vi "MultirunBuilderForNamedLocations.vi"() -> ()   [LabVIEW 2015]
uses:
  Anemometry Sub Vis/Gen Trav/Spacing.ctl
  Anemometry Sub Vis/Controls/Multi_run_mode.ctl
  Anemometry Sub Vis/File/Setup_Filetype.ctl
  Anemometry Sub Vis/Globals/Meas_global.vi
panel:
  in  "Vert.Z-Locations 2":dbl[](array[numeric])=[12.7, 19.05, 25.4]
  in  "TaskArray":T3(array[cluster])=[{"Start X"=-3390.0, "Start Y"=-113.0, "Start Z"=780.0, "End X"=-3390.0, "End Y"=-113.0, "End Z"=780.0, "No. of pts."=0, "Spacing"=enum."Linear", "Filename"=path "", "Tunnel Speed"=7.64, "Averaging time (min)"=0.0, "Extra Commands"="", "Carrier_1 Q (l/min)"=0.0, "Carrier_2 Q (l/min)"=0.0, "Trace Gas Concentration (%)"=0.0, "Specific Arguments"="", "Comments"="Tunnel Warm Up", "Row No"=0, "Row Type Selector"=enum."Set Tunnel Speed Only", "Completion time"="", "Row Duration (mins)"=10.0, "No. of Valid pts."=0, "Meas Setup File"=""}, {"Start X"=-3390.0, "Start Y"=-113.0, "Start Z"=780.0, "End X"=-3390.0, "End Y"=-113.0, "End Z"=780.0, "No. of pts."=0, "Spacing"=enum."Linear", "Filename"=path "", "Tunnel Speed"=7.64, "Averaging time (min)"=0.0, "Extra Commands"="", "Carrier_1 Q (l/min)"=0.0, "Carrier_2 Q (l/min)"=0.0, "Trace Gas Concentration (%)"=0.0, "Specific Arguments"="10", "Comments"="Tunnel Warm Up", "Row No"=0, "Row Type Selector"=enum."Wait (minutes)", "Completion time"="", "Row Duration (mins)"=0.0, "No. of Valid pts."=0, "Meas Setup File"=""}, {"Start X"=0.0, "Start Y"=0.0, "Start Z"=150.0, "End X"=0.0, "End Y"=0.0, "End Z"=150.0, "No. of pts."=0, "Spacing"=enum."Linear", "Filename"=path "", "Tunnel Speed"=7.64, "Averaging time (min)"=0.0, "Extra Commands"="!Work in Tunnel Coordinates", "Carrier_1 Q (l/min)"=0.0, "Carrier_2 Q (l/min)"=0.0, "Trace Gas Concentration (%)"=0.0, "Specific Arguments"="", "Comments"="", "Row No"=0, "Row Type Selector"=enum."Move Traverse Only", "Completion time"="", "Row Duration (mins)"=0.0, "No. of Valid pts."=0, "Meas Setup File"=""}, {"Start X"=0.0, "Start Y"=0.0, "Start Z"=805.0, "End X"=0.0, "End Y"=0.0, "End Z"=805.0, "No. of pts."=0, "Spacing"=enum."Linear", "Filename"=path "", "Tunnel Speed"=7.64, "Averaging time (min)"=0.0, "Extra Commands"="!Work in Tunnel Coordinates", "Carrier_1 Q (l/min)"=0.0, "Carrier_2 Q (l/min)"=0.0, "Trace Gas Concentration (%)"=0.0, "Specific Arguments"="MoveTT.vi;10", "Comments"="", "Row No"=0, "Row Type Selector"=enum."Run VI Named:", "Completion time"="", "Row Duration (mins)"=0.0, "No. of Valid pts."=0, "Meas Setup File"=""}, {"Start X"=-72.9, "Start Y"=-56.5, "Start Z"=12.7, "End X"=-72.9, "End Y"=-56.5, "End Z"=25.4, "No. of pts."=3, "Spacing"=enum."Specified", "Filename"=path "M:/\\Projects\\8773\\Results\\Tunnel1\\AnemometerSurvey.xls", "Tunnel Speed"=7.64, "Averaging time (min)"=1.0, "Extra Commands"="", "Carrier_1 Q (l/min)"=0.0, "Carrier_2 Q (l/min)"=0.0, "Trace Gas Concentration (%)"=0.0, "Specific Arguments"="Z= ;12.7;19.1;25.4\r", "Comments"="Anemo1", "Row No"=0, "Row Type Selector"=enum."Vertical Profile", "Completion time"="", "Row Duration (mins)"=0.0, "No. of Valid pts."=0, "Meas Setup File"="Current_Setup.xls"}, {"Start X"=-458.4, "Start Y"=87.9, "Start Z"=25.6, "End X"=-458.4, "End Y"=87.9, "End Z"=38.3, "No. of pts."=3, "Spacing"=enum."Specified", "Filename"=path "M:/\\Projects\\8773\\Results\\Tunnel1\\AnemometerSurvey.xls", "Tunnel Speed"=7.64, "Averaging time (min)"=1.0, "Extra Commands"="", "Carrier_1 Q (l/min)"=0.0, "Carrier_2 Q (l/min)"=0.0, "Trace Gas Concentration (%)"=0.0, "Specific Arguments"="Z= ;25.6;32.0;38.3\r", "Comments"="Anemo2", "Row No"=0, "Row Type Selector"=enum."Vertical Profile", "Completion time"="", "Row Duration (mins)"=0.0, "No. of Valid pts."=0, "Meas Setup File"="Current_Setup.xls"}, {"Start X"=0.0, "Start Y"=0.0, "Start Z"=150.0, "End X"=0.0, "End Y"=0.0, "End Z"=150.0, "No. of pts."=0, "Spacing"=enum."Linear", "Filename"=path "", "Tunnel Speed"=7.64, "Averaging time (min)"=0.0, "Extra Commands"="!Work in Tunnel Coordinates", "Carrier_1 Q (l/min)"=0.0, "Carrier_2 Q (l/min)"=0.0, "Trace Gas Concentration (%)"=0.0, "Specific Arguments"="", "Comments"="", "Row No"=0, "Row Type Selector"=enum."Move Traverse Only", "Completion time"="", "Row Duration (mins)"=0.0, "No. of Valid pts."=0, "Meas Setup File"=""}, {"Start X"=0.0, "Start Y"=0.0, "Start Z"=805.0, "End X"=0.0, "End Y"=0.0, "End Z"=805.0, "No. of pts."=0, "Spacing"=enum."Linear", "Filename"=path "", "Tunnel Speed"=7.64, "Averaging time (min)"=0.0, "Extra Commands"="!Work in Tunnel Coordinates", "Carrier_1 Q (l/min)"=0.0, "Carrier_2 Q (l/min)"=0.0, "Trace Gas Concentration (%)"=0.0, "Specific Arguments"="MoveTT.vi;30", "Comments"="", "Row No"=0, "Row Type Selector"=enum."Run VI Named:", "Completion time"="", "Row Duration (mins)"=0.0, "No. of Valid pts."=0, "Meas Setup File"=""}, {"Start X"=-72.9, "Start Y"=-56.5, "Start Z"=12.7, "End X"=-72.9, "End Y"=-56.5, "End Z"=25.4, "No. of pts."=3, "Spacing"=enum."Specified", "Filename"=path "M:/\\Projects\\8773\\Results\\Tunnel1\\AnemometerSurvey.xls", "Tunnel Speed"=7.64, "Averaging time (min)"=1.0, "Extra Commands"="", "Carrier_1 Q (l/min)"=0.0, "Carrier_2 Q (l/min)"=0.0, "Trace Gas Concentration (%)"=0.0, "Specific Arguments"="Z= ;12.7;19.1;25.4\r", "Comments"="Anemo1", "Row No"=0, "Row Type Selector"=enum."Vertical Profile", "Completion time"="", "Row Duration (mins)"=0.0, "No. of Valid pts."=0, "Meas Setup File"="Current_Setup.xls"}, {"Start X"=-458.4, "Start Y"=87.9, "Start Z"=25.6, "End X"=-458.4, "End Y"=87.9, "End Z"=38.3, "No. of pts."=3, "Spacing"=enum."Specified", "Filename"=path "M:/\\Projects\\8773\\Results\\Tunnel1\\AnemometerSurvey.xls", "Tunnel Speed"=7.64, "Averaging time (min)"=1.0, "Extra Commands"="", "Carrier_1 Q (l/min)"=0.0, "Carrier_2 Q (l/min)"=0.0, "Trace Gas Concentration (%)"=0.0, "Specific Arguments"="Z= ;25.6;32.0;38.3\r", "Comments"="Anemo2", "Row No"=0, "Row Type Selector"=enum."Vertical Profile", "Completion time"="", "Row Duration (mins)"=0.0, "No. of Valid pts."=0, "Meas Setup File"="Current_Setup.xls"}, {"Start X"=0.0, "Start Y"=0.0, "Start Z"=150.0, "End X"=0.0, "End Y"=0.0, "End Z"=150.0, "No. of pts."=0, "Spacing"=enum."Linear", "Filename"=path "", "Tunnel Speed"=7.64, "Averaging time (min)"=0.0, "Extra Commands"="!Work in Tunnel Coordinates", "Carrier_1 Q (l/min)"=0.0, "Carrier_2 Q (l/min)"=0.0, "Trace Gas Concentration (%)"=0.0, "Specific Arguments"="", "Comments"="", "Row No"=0, "Row Type Selector"=enum."Move Traverse Only", "Completion time"="", "Row Duration (mins)"=0.0, "No. of Valid pts."=0, "Meas Setup File"=""}, {"Start X"=0.0, "Start Y"=0.0, "Start Z"=805.0, "End X"=0.0, "End Y"=0.0, "End Z"=805.0, "No. of pts."=0, "Spacing"=enum."Linear", "Filename"=path "", "Tunnel Speed"=7.64, "Averaging time (min)"=0.0, "Extra Commands"="!Work in Tunnel Coordinates", "Carrier_1 Q (l/min)"=0.0, "Carrier_2 Q (l/min)"=0.0, "Trace Gas Concentration (%)"=0.0, "Specific Arguments"="MoveTT.vi;50", "Comments"="", "Row No"=0, "Row Type Selector"=enum."Run VI Named:", "Completion time"="", "Row Duration (mins)"=0.0, "No. of Valid pts."=0, "Meas Setup File"=""}, {"Start X"=-72.9, "Start Y"=-56.5, "Start Z"=12.7, "End X"=-72.9, "End Y"=-56.5, "End Z"=25.4, "No. of pts."=3, "Spacing"=enum."Specified", "Filename"=path "M:/\\Projects\\8773\\Results\\Tunnel1\\AnemometerSurvey.xls", "Tunnel Speed"=7.64, "Averaging time (min)"=1.0, "Extra Commands"="", "Carrier_1 Q (l/min)"=0.0, "Carrier_2 Q (l/min)"=0.0, "Trace Gas Concentration (%)"=0.0, "Specific Arguments"="Z= ;12.7;19.1;25.4\r", "Comments"="Anemo1", "Row No"=0, "Row Type Selector"=enum."Vertical Profile", "Completion time"="", "Row Duration (mins)"=0.0, "No. of Valid pts."=0, "Meas Setup File"="Current_Setup.xls"}, {"Start X"=-458.4, "Start Y"=87.9, "Start Z"=25.6, "End X"=-458.4, "End Y"=87.9, "End Z"=38.3, "No. of pts."=3, "Spacing"=enum."Specified", "Filename"=path "M:/\\Projects\\8773\\Results\\Tunnel1\\AnemometerSurvey.xls", "Tunnel Speed"=7.64, "Averaging time (min)"=1.0, "Extra Commands"="", "Carrier_1 Q (l/min)"=0.0, "Carrier_2 Q (l/min)"=0.0, "Trace Gas Concentration (%)"=0.0, "Specific Arguments"="Z= ;25.6;32.0;38.3\r", "Comments"="Anemo2", "Row No"=0, "Row Type Selector"=enum."Vertical Profile", "Completion time"="", "Row Duration (mins)"=0.0, "No. of Valid pts."=0, "Meas Setup File"="Current_Setup.xls"}, {"Start X"=0.0, "Start Y"=0.0, "Start Z"=150.0, "End X"=0.0, "End Y"=0.0, "End Z"=150.0, "No. of pts."=0, "Spacing"=enum."Linear", "Filename"=path "", "Tunnel Speed"=7.64, "Averaging time (min)"=0.0, "Extra Commands"="!Work in Tunnel Coordinates", "Carrier_1 Q (l/min)"=0.0, "Carrier_2 Q (l/min)"=0.0, "Trace Gas Concentration (%)"=0.0, "Specific Arguments"="", "Comments"="", "Row No"=0, "Row Type Selector"=enum."Move Traverse Only", "Completion time"="", "Row Duration (mins)"=0.0, "No. of Valid pts."=0, "Meas Setup File"=""}, {"Start X"=0.0, "Start Y"=0.0, "Start Z"=805.0, "End X"=0.0, "End Y"=0.0, "End Z"=805.0, "No. of pts."=0, "Spacing"=enum."Linear", "Filename"=path "", "Tunnel Speed"=7.64, "Averaging time (min)"=0.0, "Extra Commands"="!Work in Tunnel Coordinates", "Carrier_1 Q (l/min)"=0.0, "Carrier_2 Q (l/min)"=0.0, "Trace Gas Concentration (%)"=0.0, "Specific Arguments"="MoveTT.vi;70", "Comments"="", "Row No"=0, "Row Type Selector"=enum."Run VI Named:", "Completion time"="", "Row Duration (mins)"=0.0, "No. of Valid pts."=0, "Meas Setup File"=""}, {"Start X"=-72.9, "Start Y"=-56.5, "Start Z"=12.7, "End X"=-72.9, "End Y"=-56.5, "End Z"=25.4, "No. of pts."=3, "Spacing"=enum."Specified", "Filename"=path "M:/\\Projects\\8773\\Results\\Tunnel1\\AnemometerSurvey.xls", "Tunnel Speed"=7.64, "Averaging time (min)"=1.0, "Extra Commands"="", "Carrier_1 Q (l/min)"=0.0, "Carrier_2 Q (l/min)"=0.0, "Trace Gas Concentration (%)"=0.0, "Specific Arguments"="Z= ;12.7;19.1;25.4\r", "Comments"="Anemo1", "Row No"=0, "Row Type Selector"=enum."Vertical Profile", "Completion time"="", "Row Duration (mins)"=0.0, "No. of Valid pts."=0, "Meas Setup File"="Current_Setup.xls"}, {"Start X"=-458.4, "Start Y"=87.9, "Start Z"=25.6, "End X"=-458.4, "End Y"=87.9, "End Z"=38.3, "No. of pts."=3, "Spacing"=enum."Specified", "Filename"=path "M:/\\Projects\\8773\\Results\\Tunnel1\\AnemometerSurvey.xls", "Tunnel Speed"=7.64, "Averaging time (min)"=1.0, "Extra Commands"="", "Carrier_1 Q (l/min)"=0.0, "Carrier_2 Q (l/min)"=0.0, "Trace Gas Concentration (%)"=0.0, "Specific Arguments"="Z= ;25.6;32.0;38.3\r", "Comments"="Anemo2", "Row No"=0, "Row Type Selector"=enum."Vertical Profile", "Completion time"="", "Row Duration (mins)"=0.0, "No. of Valid pts."=0, "Meas Setup File"="Current_Setup.xls"}, {"Start X"=0.0, "Start Y"=0.0, "Start Z"=150.0, "End X"=0.0, "End Y"=0.0, "End Z"=150.0, "No. of pts."=0, "Spacing"=enum."Linear", "Filename"=path "", "Tunnel Speed"=7.64, "Averaging time (min)"=0.0, "Extra Commands"="!Work in Tunnel Coordinates", "Carrier_1 Q (l/min)"=0.0, "Carrier_2 Q (l/min)"=0.0, "Trace Gas Concentration (%)"=0.0, "Specific Arguments"="", "Comments"="", "Row No"=0, "Row Type Selector"=enum."Move Traverse Only", "Completion time"="", "Row Duration (mins)"=0.0, "No. of Valid pts."=0, "Meas Setup File"=""}, {"Start X"=0.0, "Start Y"=0.0, "Start Z"=805.0, "End X"=0.0, "End Y"=0.0, "End Z"=805.0, "No. of pts."=0, "Spacing"=enum."Linear", "Filename"=path "", "Tunnel Speed"=7.64, "Averaging time (min)"=0.0, "Extra Commands"="!Work in Tunnel Coordinates", "Carrier_1 Q (l/min)"=0.0, "Carrier_2 Q (l/min)"=0.0, "Trace Gas Concentration (%)"=0.0, "Specific Arguments"="MoveTT.vi;90", "Comments"="", "Row No"=0, "Row Type Selector"=enum."Run VI Named:", "Completion time"="", "Row Duration (mins)"=0.0, "No. of Valid pts."=0, "Meas Setup File"=""}, {"Start X"=-72.9, "Start Y"=-56.5, "Start Z"=12.7, "End X"=-72.9, "End Y"=-56.5, "End Z"=25.4, "No. of pts."=3, "Spacing"=enum."Specified", "Filename"=path "M:/\\Projects\\8773\\Results\\Tunnel1\\AnemometerSurvey.xls", "Tunnel Speed"=7.64, "Averaging time (min)"=1.0, "Extra Commands"="", "Carrier_1 Q (l/min)"=0.0, "Carrier_2 Q (l/min)"=0.0, "Trace Gas Concentration (%)"=0.0, "Specific Arguments"="Z= ;12.7;19.1;25.4\r", "Comments"="Anemo1", "Row No"=0, "Row Type Selector"=enum."Vertical Profile", "Completion time"="", "Row Duration (mins)"=0.0, "No. of Valid pts."=0, "Meas Setup File"="Current_Setup.xls"}, {"Start X"=-458.4, "Start Y"=87.9, "Start Z"=25.6, "End X"=-458.4, "End Y"=87.9, "End Z"=38.3, "No. of pts."=3, "Spacing"=enum."Specified", "Filename"=path "M:/\\Projects\\8773\\Results\\Tunnel1\\AnemometerSurvey.xls", "Tunnel Speed"=7.64, "Averaging time (min)"=1.0, "Extra Commands"="", "Carrier_1 Q (l/min)"=0.0, "Carrier_2 Q (l/min)"=0.0, "Trace Gas Concentration (%)"=0.0, "Specific Arguments"="Z= ;25.6;32.0;38.3\r", "Comments"="Anemo2", "Row No"=0, "Row Type Selector"=enum."Vertical Profile", "Completion time"="", "Row Duration (mins)"=0.0, "No. of Valid pts."=0, "Meas Setup File"="Current_Setup.xls"}, {"Start X"=0.0, "Start Y"=0.0, "Start Z"=150.0, "End X"=0.0, "End Y"=0.0, "End Z"=150.0, "No. of pts."=0, "Spacing"=enum."Linear", "Filename"=path "", "Tunnel Speed"=7.64, "Averaging time (min)"=0.0, "Extra Commands"="!Work in Tunnel Coordinates", "Carrier_1 Q (l/min)"=0.0, "Carrier_2 Q (l/min)"=0.0, "Trace Gas Concentration (%)"=0.0, "Specific Arguments"="", "Comments"="", "Row No"=0, "Row Type Selector"=enum."Move Traverse Only", "Completion time"="", "Row Duration (mins)"=0.0, "No. of Valid pts."=0, "Meas Setup File"=""}, {"Start X"=0.0, "Start Y"=0.0, "Start Z"=805.0, "End X"=0.0, "End Y"=0.0, "End Z"=805.0, "No. of pts."=0, "Spacing"=enum."Linear", "Filename"=path "", "Tunnel Speed"=7.64, "Averaging time (min)"=0.0, "Extra Commands"="!Work in Tunnel Coordinates", "Carrier_1 Q (l/min)"=0.0, "Carrier_2 Q (l/min)"=0.0, "Trace Gas Concentration (%)"=0.0, "Specific Arguments"="MoveTT.vi;110", "Comments"="", "Row No"=0, "Row Type Selector"=enum."Run VI Named:", "Completion time"="", "Row Duration (mins)"=0.0, "No. of Valid pts."=0, "Meas Setup File"=""}, {"Start X"=-72.9, "Start Y"=-56.5, "Start Z"=12.7, "End X"=-72.9, "End Y"=-56.5, "End Z"=25.4, "No. of pts."=3, "Spacing"=enum."Specified", "Filename"=path "M:/\\Projects\\8773\\Results\\Tunnel1\\AnemometerSurvey.xls", "Tunnel Speed"=7.64, "Averaging time (min)"=1.0, "Extra Commands"="", "Carrier_1 Q (l/min)"=0.0, "Carrier_2 Q (l/min)"=0.0, "Trace Gas Concentration (%)"=0.0, "Specific Arguments"="Z= ;12.7;19.1;25.4\r", "Comments"="Anemo1", "Row No"=0, "Row Type Selector"=enum."Vertical Profile", "Completion time"="", "Row Duration (mins)"=0.0, "No. of Valid pts."=0, "Meas Setup File"="Current_Setup.xls"}, {"Start X"=-458.4, "Start Y"=87.9, "Start Z"=25.6, "End X"=-458.4, "End Y"=87.9, "End Z"=38.3, "No. of pts."=3, "Spacing"=enum."Specified", "Filename"=path "M:/\\Projects\\8773\\Results\\Tunnel1\\AnemometerSurvey.xls", "Tunnel Speed"=7.64, "Averaging time (min)"=1.0, "Extra Commands"="", "Carrier_1 Q (l/min)"=0.0, "Carrier_2 Q (l/min)"=0.0, "Trace Gas Concentration (%)"=0.0, "Specific Arguments"="Z= ;25.6;32.0;38.3\r", "Comments"="Anemo2", "Row No"=0, "Row Type Selector"=enum."Vertical Profile", "Completion time"="", "Row Duration (mins)"=0.0, "No. of Valid pts."=0, "Meas Setup File"="Current_Setup.xls"}, {"Start X"=0.0, "Start Y"=0.0, "Start Z"=150.0, "End X"=0.0, "End Y"=0.0, "End Z"=150.0, "No. of pts."=0, "Spacing"=enum."Linear", "Filename"=path "", "Tunnel Speed"=7.64, "Averaging time (min)"=0.0, "Extra Commands"="!Work in Tunnel Coordinates", "Carrier_1 Q (l/min)"=0.0, "Carrier_2 Q (l/min)"=0.0, "Trace Gas Concentration (%)"=0.0, "Specific Arguments"="", "Comments"="", "Row No"=0, "Row Type Selector"=enum."Move Traverse Only", "Completion time"="", "Row Duration (mins)"=0.0, "No. of Valid pts."=0, "Meas Setup File"=""}, {"Start X"=0.0, "Start Y"=0.0, "Start Z"=805.0, "End X"=0.0, "End Y"=0.0, "End Z"=805.0, "No. of pts."=0, "Spacing"=enum."Linear", "Filename"=path "", "Tunnel Speed"=7.64, "Averaging time (min)"=0.0, "Extra Commands"="!Work in Tunnel Coordinates", "Carrier_1 Q (l/min)"=0.0, "Carrier_2 Q (l/min)"=0.0, "Trace Gas Concentration (%)"=0.0, "Specific Arguments"="MoveTT.vi;130", "Comments"="", "Row No"=0, "Row Type Selector"=enum."Run VI Named:", "Completion time"="", "Row Duration (mins)"=0.0, "No. of Valid pts."=0, "Meas Setup File"=""}, {"Start X"=-72.9, "Start Y"=-56.5, "Start Z"=12.7, "End X"=-72.9, "End Y"=-56.5, "End Z"=25.4, "No. of pts."=3, "Spacing"=enum."Specified", "Filename"=path "M:/\\Projects\\8773\\Results\\Tunnel1\\AnemometerSurvey.xls", "Tunnel Speed"=7.64, "Averaging time (min)"=1.0, "Extra Commands"="", "Carrier_1 Q (l/min)"=0.0, "Carrier_2 Q (l/min)"=0.0, "Trace Gas Concentration (%)"=0.0, "Specific Arguments"="Z= ;12.7;19.1;25.4\r", "Comments"="Anemo1", "Row No"=0, "Row Type Selector"=enum."Vertical Profile", "Completion time"="", "Row Duration (mins)"=0.0, "No. of Valid pts."=0, "Meas Setup File"="Current_Setup.xls"}, {"Start X"=-458.4, "Start Y"=87.9, "Start Z"=25.6, "End X"=-458.4, "End Y"=87.9, "End Z"=38.3, "No. of pts."=3, "Spacing"=enum."Specified", "Filename"=path "M:/\\Projects\\8773\\Results\\Tunnel1\\AnemometerSurvey.xls", "Tunnel Speed"=7.64, "Averaging time (min)"=1.0, "Extra Commands"="", "Carrier_1 Q (l/min)"=0.0, "Carrier_2 Q (l/min)"=0.0, "Trace Gas Concentration (%)"=0.0, "Specific Arguments"="Z= ;25.6;32.0;38.3\r", "Comments"="Anemo2", "Row No"=0, "Row Type Selector"=enum."Vertical Profile", "Completion time"="", "Row Duration (mins)"=0.0, "No. of Valid pts."=0, "Meas Setup File"="Current_Setup.xls"}, {"Start X"=0.0, "Start Y"=0.0, "Start Z"=150.0, "End X"=0.0, "End Y"=0.0, "End Z"=150.0, "No. of pts."=0, "Spacing"=enum."Linear", "Filename"=path "", "Tunnel Speed"=7.64, "Averaging time (min)"=0.0, "Extra Commands"="!Work in Tunnel Coordinates", "Carrier_1 Q (l/min)"=0.0, "Carrier_2 Q (l/min)"=0.0, "Trace Gas Concentration (%)"=0.0, "Specific Arguments"="", "Comments"="", "Row No"=0, "Row Type Selector"=enum."Move Traverse Only", "Completion time"="", "Row Duration (mins)"=0.0, "No. of Valid pts."=0, "Meas Setup File"=""}, {"Start X"=0.0, "Start Y"=0.0, "Start Z"=805.0, "End X"=0.0, "End Y"=0.0, "End Z"=805.0, "No. of pts."=0, "Spacing"=enum."Linear", "Filename"=path "", "Tunnel Speed"=7.64, "Averaging time (min)"=0.0, "Extra Commands"="!Work in Tunnel Coordinates", "Carrier_1 Q (l/min)"=0.0, "Carrier_2 Q (l/min)"=0.0, "Trace Gas Concentration (%)"=0.0, "Specific Arguments"="MoveTT.vi;150", "Comments"="", "Row No"=0, "Row Type Selector"=enum."Run VI Named:", "Completion time"="", "Row Duration (mins)"=0.0, "No. of Valid pts."=0, "Meas Setup File"=""}, {"Start X"=-72.9, "Start Y"=-56.5, "Start Z"=12.7, "End X"=-72.9, "End Y"=-56.5, "End Z"=25.4, "No. of pts."=3, "Spacing"=enum."Specified", "Filename"=path "M:/\\Projects\\8773\\Results\\Tunnel1\\AnemometerSurvey.xls", "Tunnel Speed"=7.64, "Averaging time (min)"=1.0, "Extra Commands"="", "Carrier_1 Q (l/min)"=0.0, "Carrier_2 Q (l/min)"=0.0, "Trace Gas Concentration (%)"=0.0, "Specific Arguments"="Z= ;12.7;19.1;25.4\r", "Comments"="Anemo1", "Row No"=0, "Row Type Selector"=enum."Vertical Profile", "Completion time"="", "Row Duration (mins)"=0.0, "No. of Valid pts."=0, "Meas Setup File"="Current_Setup.xls"}, {"Start X"=-458.4, "Start Y"=87.9, "Start Z"=25.6, "End X"=-458.4, "End Y"=87.9, "End Z"=38.3, "No. of pts."=3, "Spacing"=enum."Specified", "Filename"=path "M:/\\Projects\\8773\\Results\\Tunnel1\\AnemometerSurvey.xls", "Tunnel Speed"=7.64, "Averaging time (min)"=1.0, "Extra Commands"="", "Carrier_1 Q (l/min)"=0.0, "Carrier_2 Q (l/min)"=0.0, "Trace Gas Concentration (%)"=0.0, "Specific Arguments"="Z= ;25.6;32.0;38.3\r", "Comments"="Anemo2", "Row No"=0, "Row Type Selector"=enum."Vertical Profile", "Completion time"="", "Row Duration (mins)"=0.0, "No. of Valid pts."=0, "Meas Setup File"="Current_Setup.xls"}, {"Start X"=0.0, "Start Y"=0.0, "Start Z"=150.0, "End X"=0.0, "End Y"=0.0, "End Z"=150.0, "No. of pts."=0, "Spacing"=enum."Linear", "Filename"=path "", "Tunnel Speed"=7.64, "Averaging time (min)"=0.0, "Extra Commands"="!Work in Tunnel Coordinates", "Carrier_1 Q (l/min)"=0.0, "Carrier_2 Q (l/min)"=0.0, "Trace Gas Concentration (%)"=0.0, "Specific Arguments"="", "Comments"="", "Row No"=0, "Row Type Selector"=enum."Move Traverse Only", "Completion time"="", "Row Duration (mins)"=0.0, "No. of Valid pts."=0, "Meas Setup File"=""}, {"Start X"=0.0, "Start Y"=0.0, "Start Z"=805.0, "End X"=0.0, "End Y"=0.0, "End Z"=805.0, "No. of pts."=0, "Spacing"=enum."Linear", "Filename"=path "", "Tunnel Speed"=7.64, "Averaging time (min)"=0.0, "Extra Commands"="!Work in Tunnel Coordinates", "Carrier_1 Q (l/min)"=0.0, "Carrier_2 Q (l/min)"=0.0, "Trace Gas Concentration (%)"=0.0, "Specific Arguments"="MoveTT.vi;170", "Comments"="", "Row No"=0, "Row Type Selector"=enum."Run VI Named:", "Completion time"="", "Row Duration (mins)"=0.0, "No. of Valid pts."=0, "Meas Setup File"=""}, {"Start X"=-72.9, "Start Y"=-56.5, "Start Z"=12.7, "End X"=-72.9, "End Y"=-56.5, "End Z"=25.4, "No. of pts."=3, "Spacing"=enum."Specified", "Filename"=path "M:/\\Projects\\8773\\Results\\Tunnel1\\AnemometerSurvey.xls", "Tunnel Speed"=7.64, "Averaging time (min)"=1.0, "Extra Commands"="", "Carrier_1 Q (l/min)"=0.0, "Carrier_2 Q (l/min)"=0.0, "Trace Gas Concentration (%)"=0.0, "Specific Arguments"="Z= ;12.7;19.1;25.4\r", "Comments"="Anemo1", "Row No"=0, "Row Type Selector"=enum."Vertical Profile", "Completion time"="", "Row Duration (mins)"=0.0, "No. of Valid pts."=0, "Meas Setup File"="Current_Setup.xls"}, {"Start X"=-458.4, "Start Y"=87.9, "Start Z"=25.6, "End X"=-458.4, "End Y"=87.9, "End Z"=38.3, "No. of pts."=3, "Spacing"=enum."Specified", "Filename"=path "M:/\\Projects\\8773\\Results\\Tunnel1\\AnemometerSurvey.xls", "Tunnel Speed"=7.64, "Averaging time (min)"=1.0, "Extra Commands"="", "Carrier_1 Q (l/min)"=0.0, "Carrier_2 Q (l/min)"=0.0, "Trace Gas Concentration (%)"=0.0, "Specific Arguments"="Z= ;25.6;32.0;38.3\r", "Comments"="Anemo2", "Row No"=0, "Row Type Selector"=enum."Vertical Profile", "Completion time"="", "Row Duration (mins)"=0.0, "No. of Valid pts."=0, "Meas Setup File"="Current_Setup.xls"}, {"Start X"=0.0, "Start Y"=0.0, "Start Z"=150.0, "End X"=0.0, "End Y"=0.0, "End Z"=150.0, "No. of pts."=0, "Spacing"=enum."Linear", "Filename"=path "", "Tunnel Speed"=7.64, "Averaging time (min)"=0.0, "Extra Commands"="!Work in Tunnel Coordinates", "Carrier_1 Q (l/min)"=0.0, "Carrier_2 Q (l/min)"=0.0, "Trace Gas Concentration (%)"=0.0, "Specific Arguments"="", "Comments"="", "Row No"=0, "Row Type Selector"=enum."Move Traverse Only", "Completion time"="", "Row Duration (mins)"=0.0, "No. of Valid pts."=0, "Meas Setup File"=""}, {"Start X"=0.0, "Start Y"=0.0, "Start Z"=805.0, "End X"=0.0, "End Y"=0.0, "End Z"=805.0, "No. of pts."=0, "Spacing"=enum."Linear", "Filename"=path "", "Tunnel Speed"=7.64, "Averaging time (min)"=0.0, "Extra Commands"="!Work in Tunnel Coordinates", "Carrier_1 Q (l/min)"=0.0, "Carrier_2 Q (l/min)"=0.0, "Trace Gas Concentration (%)"=0.0, "Specific Arguments"="MoveTT.vi;190", "Comments"="", "Row No"=0, "Row Type Selector"=enum."Run VI Named:", "Completion time"="", "Row Duration (mins)"=0.0, "No. of Valid pts."=0, "Meas Setup File"=""}, {"Start X"=-72.9, "Start Y"=-56.5, "Start Z"=12.7, "End X"=-72.9, "End Y"=-56.5, "End Z"=25.4, "No. of pts."=3, "Spacing"=enum."Specified", "Filename"=path "M:/\\Projects\\8773\\Results\\Tunnel1\\AnemometerSurvey.xls", "Tunnel Speed"=7.64, "Averaging time (min)"=1.0, "Extra Commands"="", "Carrier_1 Q (l/min)"=0.0, "Carrier_2 Q (l/min)"=0.0, "Trace Gas Concentration (%)"=0.0, "Specific Arguments"="Z= ;12.7;19.1;25.4\r", "Comments"="Anemo1", "Row No"=0, "Row Type Selector"=enum."Vertical Profile", "Completion time"="", "Row Duration (mins)"=0.0, "No. of Valid pts."=0, "Meas Setup File"="Current_Setup.xls"}, {"Start X"=-458.4, "Start Y"=87.9, "Start Z"=25.6, "End X"=-458.4, "End Y"=87.9, "End Z"=38.3, "No. of pts."=3, "Spacing"=enum."Specified", "Filename"=path "M:/\\Projects\\8773\\Results\\Tunnel1\\AnemometerSurvey.xls", "Tunnel Speed"=7.64, "Averaging time (min)"=1.0, "Extra Commands"="", "Carrier_1 Q (l/min)"=0.0, "Carrier_2 Q (l/min)"=0.0, "Trace Gas Concentration (%)"=0.0, "Specific Arguments"="Z= ;25.6;32.0;38.3\r", "Comments"="Anemo2", "Row No"=0, "Row Type Selector"=enum."Vertical Profile", "Completion time"="", "Row Duration (mins)"=0.0, "No. of Valid pts."=0, "Meas Setup File"="Current_Setup.xls"}, {"Start X"=0.0, "Start Y"=0.0, "Start Z"=150.0, "End X"=0.0, "End Y"=0.0, "End Z"=150.0, "No. of pts."=0, "Spacing"=enum."Linear", "Filename"=path "", "Tunnel Speed"=7.64, "Averaging time (min)"=0.0, "Extra Commands"="!Work in Tunnel Coordinates", "Carrier_1 Q (l/min)"=0.0, "Carrier_2 Q (l/min)"=0.0, "Trace Gas Concentration (%)"=0.0, "Specific Arguments"="", "Comments"="", "Row No"=0, "Row Type Selector"=enum."Move Traverse Only", "Completion time"="", "Row Duration (mins)"=0.0, "No. of Valid pts."=0, "Meas Setup File"=""}, {"Start X"=0.0, "Start Y"=0.0, "Start Z"=805.0, "End X"=0.0, "End Y"=0.0, "End Z"=805.0, "No. of pts."=0, "Spacing"=enum."Linear", "Filename"=path "", "Tunnel Speed"=7.64, "Averaging time (min)"=0.0, "Extra Commands"="!Work in Tunnel Coordinates", "Carrier_1 Q (l/min)"=0.0, "Carrier_2 Q (l/min)"=0.0, "Trace Gas Concentration (%)"=0.0, "Specific Arguments"="MoveTT.vi;210", "Comments"="", "Row No"=0, "Row Type Selector"=enum."Run VI Named:", "Completion time"="", "Row Duration (mins)"=0.0, "No. of Valid pts."=0, "Meas Setup File"=""}, {"Start X"=-72.9, "Start Y"=-56.5, "Start Z"=12.7, "End X"=-72.9, "End Y"=-56.5, "End Z"=25.4, "No. of pts."=3, "Spacing"=enum."Specified", "Filename"=path "M:/\\Projects\\8773\\Results\\Tunnel1\\AnemometerSurvey.xls", "Tunnel Speed"=7.64, "Averaging time (min)"=1.0, "Extra Commands"="", "Carrier_1 Q (l/min)"=0.0, "Carrier_2 Q (l/min)"=0.0, "Trace Gas Concentration (%)"=0.0, "Specific Arguments"="Z= ;12.7;19.1;25.4\r", "Comments"="Anemo1", "Row No"=0, "Row Type Selector"=enum."Vertical Profile", "Completion time"="", "Row Duration (mins)"=0.0, "No. of Valid pts."=0, "Meas Setup File"="Current_Setup.xls"}, {"Start X"=-458.4, "Start Y"=87.9, "Start Z"=25.6, "End X"=-458.4, "End Y"=87.9, "End Z"=38.3, "No. of pts."=3, "Spacing"=enum."Specified", "Filename"=path "M:/\\Projects\\8773\\Results\\Tunnel1\\AnemometerSurvey.xls", "Tunnel Speed"=7.64, "Averaging time (min)"=1.0, "Extra Commands"="", "Carrier_1 Q (l/min)"=0.0, "Carrier_2 Q (l/min)"=0.0, "Trace Gas Concentration (%)"=0.0, "Specific Arguments"="Z= ;25.6;32.0;38.3\r", "Comments"="Anemo2", "Row No"=0, "Row Type Selector"=enum."Vertical Profile", "Completion time"="", "Row Duration (mins)"=0.0, "No. of Valid pts."=0, "Meas Setup File"="Current_Setup.xls"}, {"Start X"=0.0, "Start Y"=0.0, "Start Z"=150.0, "End X"=0.0, "End Y"=0.0, "End Z"=150.0, "No. of pts."=0, "Spacing"=enum."Linear", "Filename"=path "", "Tunnel Speed"=7.64, "Averaging time (min)"=0.0, "Extra Commands"="!Work in Tunnel Coordinates", "Carrier_1 Q (l/min)"=0.0, "Carrier_2 Q (l/min)"=0.0, "Trace Gas Concentration (%)"=0.0, "Specific Arguments"="", "Comments"="", "Row No"=0, "Row Type Selector"=enum."Move Traverse Only", "Completion time"="", "Row Duration (mins)"=0.0, "No. of Valid pts."=0, "Meas Setup File"=""}, {"Start X"=0.0, "Start Y"=0.0, "Start Z"=805.0, "End X"=0.0, "End Y"=0.0, "End Z"=805.0, "No. of pts."=0, "Spacing"=enum."Linear", "Filename"=path "", "Tunnel Speed"=7.64, "Averaging time (min)"=0.0, "Extra Commands"="!Work in Tunnel Coordinates", "Carrier_1 Q (l/min)"=0.0, "Carrier_2 Q (l/min)"=0.0, "Trace Gas Concentration (%)"=0.0, "Specific Arguments"="MoveTT.vi;230", "Comments"="", "Row No"=0, "Row Type Selector"=enum."Run VI Named:", "Completion time"="", "Row Duration (mins)"=0.0, "No. of Valid pts."=0, "Meas Setup File"=""}, {"Start X"=-72.9, "Start Y"=-56.5, "Start Z"=12.7, "End X"=-72.9, "End Y"=-56.5, "End Z"=25.4, "No. of pts."=3, "Spacing"=enum."Specified", "Filename"=path "M:/\\Projects\\8773\\Results\\Tunnel1\\AnemometerSurvey.xls", "Tunnel Speed"=7.64, "Averaging time (min)"=1.0, "Extra Commands"="", "Carrier_1 Q (l/min)"=0.0, "Carrier_2 Q (l/min)"=0.0, "Trace Gas Concentration (%)"=0.0, "Specific Arguments"="Z= ;12.7;19.1;25.4\r", "Comments"="Anemo1", "Row No"=0, "Row Type Selector"=enum."Vertical Profile", "Completion time"="", "Row Duration (mins)"=0.0, "No. of Valid pts."=0, "Meas Setup File"="Current_Setup.xls"}, {"Start X"=-458.4, "Start Y"=87.9, "Start Z"=25.6, "End X"=-458.4, "End Y"=87.9, "End Z"=38.3, "No. of pts."=3, "Spacing"=enum."Specified", "Filename"=path "M:/\\Projects\\8773\\Results\\Tunnel1\\AnemometerSurvey.xls", "Tunnel Speed"=7.64, "Averaging time (min)"=1.0, "Extra Commands"="", "Carrier_1 Q (l/min)"=0.0, "Carrier_2 Q (l/min)"=0.0, "Trace Gas Concentration (%)"=0.0, "Specific Arguments"="Z= ;25.6;32.0;38.3\r", "Comments"="Anemo2", "Row No"=0, "Row Type Selector"=enum."Vertical Profile", "Completion time"="", "Row Duration (mins)"=0.0, "No. of Valid pts."=0, "Meas Setup File"="Current_Setup.xls"}, {"Start X"=0.0, "Start Y"=0.0, "Start Z"=150.0, "End X"=0.0, "End Y"=0.0, "End Z"=150.0, "No. of pts."=0, "Spacing"=enum."Linear", "Filename"=path "", "Tunnel Speed"=7.64, "Averaging time (min)"=0.0, "Extra Commands"="!Work in Tunnel Coordinates", "Carrier_1 Q (l/min)"=0.0, "Carrier_2 Q (l/min)"=0.0, "Trace Gas Concentration (%)"=0.0, "Specific Arguments"="", "Comments"="", "Row No"=0, "Row Type Selector"=enum."Move Traverse Only", "Completion time"="", "Row Duration (mins)"=0.0, "No. of Valid pts."=0, "Meas Setup File"=""}, {"Start X"=0.0, "Start Y"=0.0, "Start Z"=805.0, "End X"=0.0, "End Y"=0.0, "End Z"=805.0, "No. of pts."=0, "Spacing"=enum."Linear", "Filename"=path "", "Tunnel Speed"=7.64, "Averaging time (min)"=0.0, "Extra Commands"="!Work in Tunnel Coordinates", "Carrier_1 Q (l/min)"=0.0, "Carrier_2 Q (l/min)"=0.0, "Trace Gas Concentration (%)"=0.0, "Specific Arguments"="MoveTT.vi;250", "Comments"="", "Row No"=0, "Row Type Selector"=enum."Run VI Named:", "Completion time"="", "Row Duration (mins)"=0.0, "No. of Valid pts."=0, "Meas Setup File"=""}, {"Start X"=-72.9, "Start Y"=-56.5, "Start Z"=12.7, "End X"=-72.9, "End Y"=-56.5, "End Z"=25.4, "No. of pts."=3, "Spacing"=enum."Specified", "Filename"=path "M:/\\Projects\\8773\\Results\\Tunnel1\\AnemometerSurvey.xls", "Tunnel Speed"=7.64, "Averaging time (min)"=1.0, "Extra Commands"="", "Carrier_1 Q (l/min)"=0.0, "Carrier_2 Q (l/min)"=0.0, "Trace Gas Concentration (%)"=0.0, "Specific Arguments"="Z= ;12.7;19.1;25.4\r", "Comments"="Anemo1", "Row No"=0, "Row Type Selector"=enum."Vertical Profile", "Completion time"="", "Row Duration (mins)"=0.0, "No. of Valid pts."=0, "Meas Setup File"="Current_Setup.xls"}, {"Start X"=-458.4, "Start Y"=87.9, "Start Z"=25.6, "End X"=-458.4, "End Y"=87.9, "End Z"=38.3, "No. of pts."=3, "Spacing"=enum."Specified", "Filename"=path "M:/\\Projects\\8773\\Results\\Tunnel1\\AnemometerSurvey.xls", "Tunnel Speed"=7.64, "Averaging time (min)"=1.0, "Extra Commands"="", "Carrier_1 Q (l/min)"=0.0, "Carrier_2 Q (l/min)"=0.0, "Trace Gas Concentration (%)"=0.0, "Specific Arguments"="Z= ;25.6;32.0;38.3\r", "Comments"="Anemo2", "Row No"=0, "Row Type Selector"=enum."Vertical Profile", "Completion time"="", "Row Duration (mins)"=0.0, "No. of Valid pts."=0, "Meas Setup File"="Current_Setup.xls"}, {"Start X"=0.0, "Start Y"=0.0, "Start Z"=150.0, "End X"=0.0, "End Y"=0.0, "End Z"=150.0, "No. of pts."=0, "Spacing"=enum."Linear", "Filename"=path "", "Tunnel Speed"=7.64, "Averaging time (min)"=0.0, "Extra Commands"="!Work in Tunnel Coordinates", "Carrier_1 Q (l/min)"=0.0, "Carrier_2 Q (l/min)"=0.0, "Trace Gas Concentration (%)"=0.0, "Specific Arguments"="", "Comments"="", "Row No"=0, "Row Type Selector"=enum."Move Traverse Only", "Completion time"="", "Row Duration (mins)"=0.0, "No. of Valid pts."=0, "Meas Setup File"=""}, {"Start X"=0.0, "Start Y"=0.0, "Start Z"=805.0, "End X"=0.0, "End Y"=0.0, "End Z"=805.0, "No. of pts."=0, "Spacing"=enum."Linear", "Filename"=path "", "Tunnel Speed"=7.64, "Averaging time (min)"=0.0, "Extra Commands"="!Work in Tunnel Coordinates", "Carrier_1 Q (l/min)"=0.0, "Carrier_2 Q (l/min)"=0.0, "Trace Gas Concentration (%)"=0.0, "Specific Arguments"="MoveTT.vi;270", "Comments"="", "Row No"=0, "Row Type Selector"=enum."Run VI Named:", "Completion time"="", "Row Duration (mins)"=0.0, "No. of Valid pts."=0, "Meas Setup File"=""}, {"Start X"=-72.9, "Start Y"=-56.5, "Start Z"=12.7, "End X"=-72.9, "End Y"=-56.5, "End Z"=25.4, "No. of pts."=3, "Spacing"=enum."Specified", "Filename"=path "M:/\\Projects\\8773\\Results\\Tunnel1\\AnemometerSurvey.xls", "Tunnel Speed"=7.64, "Averaging time (min)"=1.0, "Extra Commands"="", "Carrier_1 Q (l/min)"=0.0, "Carrier_2 Q (l/min)"=0.0, "Trace Gas Concentration (%)"=0.0, "Specific Arguments"="Z= ;12.7;19.1;25.4\r", "Comments"="Anemo1", "Row No"=0, "Row Type Selector"=enum."Vertical Profile", "Completion time"="", "Row Duration (mins)"=0.0, "No. of Valid pts."=0, "Meas Setup File"="Current_Setup.xls"}, {"Start X"=-458.4, "Start Y"=87.9, "Start Z"=25.6, "End X"=-458.4, "End Y"=87.9, "End Z"=38.3, "No. of pts."=3, "Spacing"=enum."Specified", "Filename"=path "M:/\\Projects\\8773\\Results\\Tunnel1\\AnemometerSurvey.xls", "Tunnel Speed"=7.64, "Averaging time (min)"=1.0, "Extra Commands"="", "Carrier_1 Q (l/min)"=0.0, "Carrier_2 Q (l/min)"=0.0, "Trace Gas Concentration (%)"=0.0, "Specific Arguments"="Z= ;25.6;32.0;38.3\r", "Comments"="Anemo2", "Row No"=0, "Row Type Selector"=enum."Vertical Profile", "Completion time"="", "Row Duration (mins)"=0.0, "No. of Valid pts."=0, "Meas Setup File"="Current_Setup.xls"}, {"Start X"=0.0, "Start Y"=0.0, "Start Z"=150.0, "End X"=0.0, "End Y"=0.0, "End Z"=150.0, "No. of pts."=0, "Spacing"=enum."Linear", "Filename"=path "", "Tunnel Speed"=7.64, "Averaging time (min)"=0.0, "Extra Commands"="!Work in Tunnel Coordinates", "Carrier_1 Q (l/min)"=0.0, "Carrier_2 Q (l/min)"=0.0, "Trace Gas Concentration (%)"=0.0, "Specific Arguments"="", "Comments"="", "Row No"=0, "Row Type Selector"=enum."Move Traverse Only", "Completion time"="", "Row Duration (mins)"=0.0, "No. of Valid pts."=0, "Meas Setup File"=""}, {"Start X"=0.0, "Start Y"=0.0, "Start Z"=805.0, "End X"=0.0, "End Y"=0.0, "End Z"=805.0, "No. of pts."=0, "Spacing"=enum."Linear", "Filename"=path "", "Tunnel Speed"=7.64, "Averaging time (min)"=0.0, "Extra Commands"="!Work in Tunnel Coordinates", "Carrier_1 Q (l/min)"=0.0, "Carrier_2 Q (l/min)"=0.0, "Trace Gas Concentration (%)"=0.0, "Specific Arguments"="MoveTT.vi;290", "Comments"="", "Row No"=0, "Row Type Selector"=enum."Run VI Named:", "Completion time"="", "Row Duration (mins)"=0.0, "No. of Valid pts."=0, "Meas Setup File"=""}, {"Start X"=-72.9, "Start Y"=-56.5, "Start Z"=12.7, "End X"=-72.9, "End Y"=-56.5, "End Z"=25.4, "No. of pts."=3, "Spacing"=enum."Specified", "Filename"=path "M:/\\Projects\\8773\\Results\\Tunnel1\\AnemometerSurvey.xls", "Tunnel Speed"=7.64, "Averaging time (min)"=1.0, "Extra Commands"="", "Carrier_1 Q (l/min)"=0.0, "Carrier_2 Q (l/min)"=0.0, "Trace Gas Concentration (%)"=0.0, "Specific Arguments"="Z= ;12.7;19.1;25.4\r", "Comments"="Anemo1", "Row No"=0, "Row Type Selector"=enum."Vertical Profile", "Completion time"="", "Row Duration (mins)"=0.0, "No. of Valid pts."=0, "Meas Setup File"="Current_Setup.xls"}, {"Start X"=-458.4, "Start Y"=87.9, "Start Z"=25.6, "End X"=-458.4, "End Y"=87.9, "End Z"=38.3, "No. of pts."=3, "Spacing"=enum."Specified", "Filename"=path "M:/\\Projects\\8773\\Results\\Tunnel1\\AnemometerSurvey.xls", "Tunnel Speed"=7.64, "Averaging time (min)"=1.0, "Extra Commands"="", "Carrier_1 Q (l/min)"=0.0, "Carrier_2 Q (l/min)"=0.0, "Trace Gas Concentration (%)"=0.0, "Specific Arguments"="Z= ;25.6;32.0;38.3\r", "Comments"="Anemo2", "Row No"=0, "Row Type Selector"=enum."Vertical Profile", "Completion time"="", "Row Duration (mins)"=0.0, "No. of Valid pts."=0, "Meas Setup File"="Current_Setup.xls"}, {"Start X"=0.0, "Start Y"=0.0, "Start Z"=150.0, "End X"=0.0, "End Y"=0.0, "End Z"=150.0, "No. of pts."=0, "Spacing"=enum."Linear", "Filename"=path "", "Tunnel Speed"=7.64, "Averaging time (min)"=0.0, "Extra Commands"="!Work in Tunnel Coordinates", "Carrier_1 Q (l/min)"=0.0, "Carrier_2 Q (l/min)"=0.0, "Trace Gas Concentration (%)"=0.0, "Specific Arguments"="", "Comments"="", "Row No"=0, "Row Type Selector"=enum."Move Traverse Only", "Completion time"="", "Row Duration (mins)"=0.0, "No. of Valid pts."=0, "Meas Setup File"=""}, {"Start X"=0.0, "Start Y"=0.0, "Start Z"=805.0, "End X"=0.0, "End Y"=0.0, "End Z"=805.0, "No. of pts."=0, "Spacing"=enum."Linear", "Filename"=path "", "Tunnel Speed"=7.64, "Averaging time (min)"=0.0, "Extra Commands"="!Work in Tunnel Coordinates", "Carrier_1 Q (l/min)"=0.0, "Carrier_2 Q (l/min)"=0.0, "Trace Gas Concentration (%)"=0.0, "Specific Arguments"="MoveTT.vi;310", "Comments"="", "Row No"=0, "Row Type Selector"=enum."Run VI Named:", "Completion time"="", "Row Duration (mins)"=0.0, "No. of Valid pts."=0, "Meas Setup File"=""}, {"Start X"=-72.9, "Start Y"=-56.5, "Start Z"=12.7, "End X"=-72.9, "End Y"=-56.5, "End Z"=25.4, "No. of pts."=3, "Spacing"=enum."Specified", "Filename"=path "M:/\\Projects\\8773\\Results\\Tunnel1\\AnemometerSurvey.xls", "Tunnel Speed"=7.64, "Averaging time (min)"=1.0, "Extra Commands"="", "Carrier_1 Q (l/min)"=0.0, "Carrier_2 Q (l/min)"=0.0, "Trace Gas Concentration (%)"=0.0, "Specific Arguments"="Z= ;12.7;19.1;25.4\r", "Comments"="Anemo1", "Row No"=0, "Row Type Selector"=enum."Vertical Profile", "Completion time"="", "Row Duration (mins)"=0.0, "No. of Valid pts."=0, "Meas Setup File"="Current_Setup.xls"}, {"Start X"=-458.4, "Start Y"=87.9, "Start Z"=25.6, "End X"=-458.4, "End Y"=87.9, "End Z"=38.3, "No. of pts."=3, "Spacing"=enum."Specified", "Filename"=path "M:/\\Projects\\8773\\Results\\Tunnel1\\AnemometerSurvey.xls", "Tunnel Speed"=7.64, "Averaging time (min)"=1.0, "Extra Commands"="", "Carrier_1 Q (l/min)"=0.0, "Carrier_2 Q (l/min)"=0.0, "Trace Gas Concentration (%)"=0.0, "Specific Arguments"="Z= ;25.6;32.0;38.3\r", "Comments"="Anemo2", "Row No"=0, "Row Type Selector"=enum."Vertical Profile", "Completion time"="", "Row Duration (mins)"=0.0, "No. of Valid pts."=0, "Meas Setup File"="Current_Setup.xls"}, {"Start X"=0.0, "Start Y"=0.0, "Start Z"=150.0, "End X"=0.0, "End Y"=0.0, "End Z"=150.0, "No. of pts."=0, "Spacing"=enum."Linear", "Filename"=path "", "Tunnel Speed"=7.64, "Averaging time (min)"=0.0, "Extra Commands"="!Work in Tunnel Coordinates", "Carrier_1 Q (l/min)"=0.0, "Carrier_2 Q (l/min)"=0.0, "Trace Gas Concentration (%)"=0.0, "Specific Arguments"="", "Comments"="", "Row No"=0, "Row Type Selector"=enum."Move Traverse Only", "Completion time"="", "Row Duration (mins)"=0.0, "No. of Valid pts."=0, "Meas Setup File"=""}, {"Start X"=0.0, "Start Y"=0.0, "Start Z"=805.0, "End X"=0.0, "End Y"=0.0, "End Z"=805.0, "No. of pts."=0, "Spacing"=enum."Linear", "Filename"=path "", "Tunnel Speed"=7.64, "Averaging time (min)"=0.0, "Extra Commands"="!Work in Tunnel Coordinates", "Carrier_1 Q (l/min)"=0.0, "Carrier_2 Q (l/min)"=0.0, "Trace Gas Concentration (%)"=0.0, "Specific Arguments"="MoveTT.vi;330", "Comments"="", "Row No"=0, "Row Type Selector"=enum."Run VI Named:", "Completion time"="", "Row Duration (mins)"=0.0, "No. of Valid pts."=0, "Meas Setup File"=""}, {"Start X"=-72.9, "Start Y"=-56.5, "Start Z"=12.7, "End X"=-72.9, "End Y"=-56.5, "End Z"=25.4, "No. of pts."=3, "Spacing"=enum."Specified", "Filename"=path "M:/\\Projects\\8773\\Results\\Tunnel1\\AnemometerSurvey.xls", "Tunnel Speed"=7.64, "Averaging time (min)"=1.0, "Extra Commands"="", "Carrier_1 Q (l/min)"=0.0, "Carrier_2 Q (l/min)"=0.0, "Trace Gas Concentration (%)"=0.0, "Specific Arguments"="Z= ;12.7;19.1;25.4\r", "Comments"="Anemo1", "Row No"=0, "Row Type Selector"=enum."Vertical Profile", "Completion time"="", "Row Duration (mins)"=0.0, "No. of Valid pts."=0, "Meas Setup File"="Current_Setup.xls"}, {"Start X"=-458.4, "Start Y"=87.9, "Start Z"=25.6, "End X"=-458.4, "End Y"=87.9, "End Z"=38.3, "No. of pts."=3, "Spacing"=enum."Specified", "Filename"=path "M:/\\Projects\\8773\\Results\\Tunnel1\\AnemometerSurvey.xls", "Tunnel Speed"=7.64, "Averaging time (min)"=1.0, "Extra Commands"="", "Carrier_1 Q (l/min)"=0.0, "Carrier_2 Q (l/min)"=0.0, "Trace Gas Concentration (%)"=0.0, "Specific Arguments"="Z= ;25.6;32.0;38.3\r", "Comments"="Anemo2", "Row No"=0, "Row Type Selector"=enum."Vertical Profile", "Completion time"="", "Row Duration (mins)"=0.0, "No. of Valid pts."=0, "Meas Setup File"="Current_Setup.xls"}, {"Start X"=0.0, "Start Y"=0.0, "Start Z"=150.0, "End X"=0.0, "End Y"=0.0, "End Z"=150.0, "No. of pts."=0, "Spacing"=enum."Linear", "Filename"=path "", "Tunnel Speed"=7.64, "Averaging time (min)"=0.0, "Extra Commands"="!Work in Tunnel Coordinates", "Carrier_1 Q (l/min)"=0.0, "Carrier_2 Q (l/min)"=0.0, "Trace Gas Concentration (%)"=0.0, "Specific Arguments"="", "Comments"="", "Row No"=0, "Row Type Selector"=enum."Move Traverse Only", "Completion time"="", "Row Duration (mins)"=0.0, "No. of Valid pts."=0, "Meas Setup File"=""}, {"Start X"=0.0, "Start Y"=0.0, "Start Z"=805.0, "End X"=0.0, "End Y"=0.0, "End Z"=805.0, "No. of pts."=0, "Spacing"=enum."Linear", "Filename"=path "", "Tunnel Speed"=7.64, "Averaging time (min)"=0.0, "Extra Commands"="!Work in Tunnel Coordinates", "Carrier_1 Q (l/min)"=0.0, "Carrier_2 Q (l/min)"=0.0, "Trace Gas Concentration (%)"=0.0, "Specific Arguments"="MoveTT.vi;350", "Comments"="", "Row No"=0, "Row Type Selector"=enum."Run VI Named:", "Completion time"="", "Row Duration (mins)"=0.0, "No. of Valid pts."=0, "Meas Setup File"=""}, {"Start X"=-72.9, "Start Y"=-56.5, "Start Z"=12.7, "End X"=-72.9, "End Y"=-56.5, "End Z"=25.4, "No. of pts."=3, "Spacing"=enum."Specified", "Filename"=path "M:/\\Projects\\8773\\Results\\Tunnel1\\AnemometerSurvey.xls", "Tunnel Speed"=7.64, "Averaging time (min)"=1.0, "Extra Commands"="", "Carrier_1 Q (l/min)"=0.0, "Carrier_2 Q (l/min)"=0.0, "Trace Gas Concentration (%)"=0.0, "Specific Arguments"="Z= ;12.7;19.1;25.4\r", "Comments"="Anemo1", "Row No"=0, "Row Type Selector"=enum."Vertical Profile", "Completion time"="", "Row Duration (mins)"=0.0, "No. of Valid pts."=0, "Meas Setup File"="Current_Setup.xls"}, {"Start X"=-458.4, "Start Y"=87.9, "Start Z"=25.6, "End X"=-458.4, "End Y"=87.9, "End Z"=38.3, "No. of pts."=3, "Spacing"=enum."Specified", "Filename"=path "M:/\\Projects\\8773\\Results\\Tunnel1\\AnemometerSurvey.xls", "Tunnel Speed"=7.64, "Averaging time (min)"=1.0, "Extra Commands"="", "Carrier_1 Q (l/min)"=0.0, "Carrier_2 Q (l/min)"=0.0, "Trace Gas Concentration (%)"=0.0, "Specific Arguments"="Z= ;25.6;32.0;38.3\r", "Comments"="Anemo2", "Row No"=0, "Row Type Selector"=enum."Vertical Profile", "Completion time"="", "Row Duration (mins)"=0.0, "No. of Valid pts."=0, "Meas Setup File"="Current_Setup.xls"}, {"Start X"=0.0, "Start Y"=0.0, "Start Z"=805.0, "End X"=0.0, "End Y"=0.0, "End Z"=805.0, "No. of pts."=0, "Spacing"=enum."Linear", "Filename"=path "", "Tunnel Speed"=7.64, "Averaging time (min)"=0.0, "Extra Commands"="!Work in Tunnel Coordinates", "Carrier_1 Q (l/min)"=0.0, "Carrier_2 Q (l/min)"=0.0, "Trace Gas Concentration (%)"=0.0, "Specific Arguments"="MoveTT.vi;0.000000", "Comments"="", "Row No"=0, "Row Type Selector"=enum."Run VI Named:", "Completion time"="", "Row Duration (mins)"=0.0, "No. of Valid pts."=0, "Meas Setup File"=""}, {"Start X"=-3390.0, "Start Y"=-113.0, "Start Z"=780.0, "End X"=-3390.0, "End Y"=-113.0, "End Z"=780.0, "No. of pts."=0, "Spacing"=enum."Linear", "Filename"=path "M:/\\Projects\\8773\\Results\\Tunnel1\\AnemometerSurvey.xls", "Tunnel Speed"=0.0, "Averaging time (min)"=1.0, "Extra Commands"="!Work in Tunnel Coordinates", "Carrier_1 Q (l/min)"=0.0, "Carrier_2 Q (l/min)"=0.0, "Trace Gas Concentration (%)"=0.0, "Specific Arguments"="", "Comments"="Zeroes", "Row No"=0, "Row Type Selector"=enum."Single Measurement", "Completion time"="", "Row Duration (mins)"=0.0, "No. of Valid pts."=0, "Meas Setup File"="Current_Setup.xls"}, {"Start X"=-3390.0, "Start Y"=-113.0, "Start Z"=780.0, "End X"=-3390.0, "End Y"=-113.0, "End Z"=780.0, "No. of pts."=0, "Spacing"=enum."Linear", "Filename"=path "M:/\\Projects\\8773\\Results\\Tunnel1\\AnemometerSurvey.xls", "Tunnel Speed"=7.64, "Averaging time (min)"=1.0, "Extra Commands"="!Work in Tunnel Coordinates", "Carrier_1 Q (l/min)"=0.0, "Carrier_2 Q (l/min)"=0.0, "Trace Gas Concentration (%)"=0.0, "Specific Arguments"="", "Comments"="CalCheck", "Row No"=0, "Row Type Selector"=enum."Single Measurement", "Completion time"="", "Row Duration (mins)"=0.0, "No. of Valid pts."=0, "Meas Setup File"="Current_Setup.xls"}, {"Start X"=0.0, "Start Y"=0.0, "Start Z"=805.0, "End X"=0.0, "End Y"=0.0, "End Z"=805.0, "No. of pts."=0, "Spacing"=enum."Linear", "Filename"=path "M:/\\Projects\\8773\\Results\\Tunnel1\\AnemometerSurvey.xls", "Tunnel Speed"=7.64, "Averaging time (min)"=1.0, "Extra Commands"="!Work in Tunnel Coordinates", "Carrier_1 Q (l/min)"=0.0, "Carrier_2 Q (l/min)"=0.0, "Trace Gas Concentration (%)"=0.0, "Specific Arguments"="", "Comments"="Local CalCheck", "Row No"=0, "Row Type Selector"=enum."Single Measurement", "Completion time"="", "Row Duration (mins)"=0.0, "No. of Valid pts."=0, "Meas Setup File"="Current_Setup.xls"}, {"Start X"=-3390.0, "Start Y"=-113.0, "Start Z"=780.0, "End X"=-3390.0, "End Y"=-113.0, "End Z"=780.0, "No. of pts."=0, "Spacing"=enum."Linear", "Filename"=path "", "Tunnel Speed"=0.0, "Averaging time (min)"=0.0, "Extra Commands"="", "Carrier_1 Q (l/min)"=0.0, "Carrier_2 Q (l/min)"=0.0, "Trace Gas Concentration (%)"=0.0, "Specific Arguments"="", "Comments"="Tunnel Off", "Row No"=0, "Row Type Selector"=enum."Set Tunnel Speed Only", "Completion time"="", "Row Duration (mins)"=0.0, "No. of Valid pts."=0, "Meas Setup File"=""}] {"Carrier_2 Q (l/min)" format="%#.2f"; "Row Duration (mins)" format="%#.1f"; "Row No" min=0; "Trace Gas Concentration (%)" min=0.0 format="%#_4f"; "Carrier_1 Q (l/min)" format="%#.2f"; "Tunnel Speed" format="%#.2f"; "Start X" format="%#.2f"; "Start Y" format="%#.2f"; "Start Z" format="%#.2f"; "End X" format="%#.2f"; "End Y" format="%#.2f"; "End Z" format="%#.2f"; "Averaging time (min)" min=0.0 format="%#.2f"}
  in  "Tab Control":T4(tab)
  in  "Command File Path / Name":path=path "/CentralDataCache/Projects/9999/Commands/Post_Processing_Machine/AnemometerSurvey.xls"
  in  "Results File Path / Name":path=path "/CentralDataCache/Projects/9999/Results/Post_Processing_Machine/AnemometerSurvey.xls"
  in  "Setup:":string(combo)="Current_Setup.xls"
  in  "Tunnel Warmup (min)":dbl=10.0
  in  "Velocity (m/s)":dbl=7.64
  in  "Measure (seconds)":dbl=60.0
  out "Measure (mins)":dbl=1.0
  in  "Multirun Closure Tasks":T5={"Turn Table --> Zero"=TRUE, "AutoCal"=FALSE, "Zeroes"=TRUE, "Global Cal Checks"=TRUE, "Local Cal Checks"=TRUE, "Tunnel Off"=TRUE}
  in  "Task Selection":T6={"Tunnel Warm Up"=TRUE, "AutoCal"=FALSE, "Zeroes"=TRUE, "Turn Table Schedule"=TRUE, "Global Cal Checks"=TRUE, "Local Cal Checks"=TRUE, "Vertical Profile"=TRUE, "Lateral Profile"=FALSE, "Reinitialize Task Array"=TRUE, "Save Command File"=TRUE, "Longitudinal Profile"=FALSE}
  in  "Zeroes":T7={"X"=-3390.0, "Y"=-113.0, "Z"=780.0, "Use Tunnel Coords?"=TRUE, "RepeatEveryXDeg"=120.0}
  in  "Local Calcheck":T8={"X"=0.0, "Y"=0.0, "Z"=805.0, "Use Tunnel Coords? Coords"=TRUE, "RepeatEveryXDeg"=60.0}
  in  "Global Calcheck":T7={"X"=-3390.0, "Y"=-113.0, "Z"=780.0, "Use Tunnel Coords?"=TRUE, "RepeatEveryXDeg"=120.0}
  in  "Message":string
  in  "Send Message after TT move?":bool=TRUE
  in  "Wait Time (min)":dbl=1440.0
  in  "Wait after TT move?":bool=TRUE
  in  "MoveTravAfterTT":T9={"X"=10.0, "Y"=10.0, "Z"=1010.0, "Use Tunnel Coords?"=TRUE, "Use Move?"=FALSE} caption="Safety Move : Move Trav After MoveTT?"
  in  "MoveTravBeforeTT":T9={"X"=0.0, "Y"=0.0, "Z"=150.0, "Use Tunnel Coords?"=TRUE, "Use Move?"=TRUE} caption="Safety Move : Move Trav Before MoveTT?"
  in  "Calculate TT Array":bool=TRUE
  in  "Angle Increment":dbl=20.0
  in  "Ending Angle":dbl=340.0
  in  "Starting Angle":dbl
  in  "Azimuth Values":dbl[](array[numeric])=[0.0, 20.0, 40.0, 60.0, 80.0, 100.0, 120.0, 140.0, 160.0, 180.0, 200.0, 220.0, 240.0, 260.0, 280.0, 300.0, 320.0, 340.0]
  in  "Vert.Z-Locations":dbl[](array[numeric])=[12.7, 19.05, 25.4]
  in  "VertProf.Coords":T10(array[cluster])=[{"X"=-72.9, "Y"=-56.5, "Z0"=0.0, "Name"="Anemo1"}, {"X"=-458.4, "Y"=87.9, "Z0"=12.9, "Name"="Anemo2"}]
  in  "VP.TTHeightCorrs":T11={"TT.Azimuths"=[0.0, 20.0, 40.0, 60.0, 80.0, 100.0, 120.0, 140.0, 160.0, 180.0, 200.0, 220.0, 240.0, 260.0, 280.0, 300.0, 320.0, 340.0], "Z.HeightCorrs"=[[-0.0, -0.0], [-0.5, -1.4000000000000057], [-1.0, -3.1000000000000085], [-0.5, -4.1000000000000085], [-0.7999999999999972, -4.900000000000006], [-0.8999999999999915, -5.6000000000000085], [-0.3999999999999915, -5.5], [0.10000000000000853, -5.1000000000000085], [0.10000000000000853, -4.700000000000003], [0.5, -3.9000000000000057], [0.6000000000000085, -2.700000000000003], [0.10000000000000853, -2.1000000000000085], [0.6000000000000085, -0.9000000000000057], [0.6000000000000085, 0.29999999999999716], [0.29999999999999716, 0.8999999999999915], [0.7999999999999972, 1.7999999999999972], [0.7000000000000028, 2.200000000000003], [-0.0, 1.2000000000000028]], "Use Height Corrections"=TRUE, "Height Survey Filepaths"=[path "/CentralDataCache/Projects/8773/Results/Tunnel1/Height Survey & Corrections/Zsurvey-Anemo1.xls", path "/CentralDataCache/Projects/8773/Results/Tunnel1/Height Survey & Corrections/Zsurvey-Anemo2.xls"], "Corrections from File"=TRUE}
  in  "Correction Channel Name":string="T1:Z:Corrections"
  in  "LatProf.Coords":T12(array[cluster])=[{"X"=1900.0, "Y0"=-500.0, "Z"=229.0, "Name"="TTLE"}, {"X"=0.0, "Y0"=-500.0, "Z"=229.0, "Name"="TTC"}, {"X"=1475.0, "Y0"=-500.0, "Z"=229.0, "Name"="TTTE"}]
  in  "Lat.Y-Locations":dbl[](array[numeric])=[-500.0, -400.0, -300.0, -200.0, -100.0, 0.0, 100.0, 200.0, 300.0, 400.0, 500.0]
  in  "Lat.HeightCorrs":T13={"Yvalues"=[0.0, 10.0, 20.0, 30.0, 40.0, 50.0, 60.0, 70.0, 80.0, 90.0, 100.0, 110.0, 120.0, 130.0, 140.0, 150.0, 160.0, 170.0, 180.0, 190.0, 200.0, 210.0, 220.0, 230.0, 240.0, 250.0, 260.0, 270.0, 280.0, 290.0, 300.0, 310.0, 320.0, 330.0, 340.0, 350.0], "X.HeightCorrs"=[[0.0], [-0.4], [-0.4], [-0.1], [0.6], [1.1], [1.5], [1.6], [1.5], [1.1], [0.3], [0.0], [-0.3], [-0.3], [-0.4], [0.7], [0.9], [1.8], [2.4], [2.5], [2.5], [2.2], [1.3], [0.7], [0.4], [0.0], [0.0], [0.8], [1.1], [1.7], [2.4], [2.4], [2.3], [2.3], [1.2], [0.4]], "Use Height Corrections"=FALSE}
  in  "LongProf.Coords":T14(array[cluster])=[{"X0"=1900.0, "Y"=-500.0, "Z"=229.0, "Name"="Window"}, {"X0"=0.0, "Y"=0.0, "Z"=229.0, "Name"="MidSpan"}, {"X0"=1475.0, "Y"=500.0, "Z"=229.0, "Name"="Wall"}]
  in  "Long.X-Locations":dbl[](array[numeric])=[-500.0, -250.0, 0.0, 250.0, 500.0]
  in  "Long.HeightCorrs":T15={"XValues"=[0.0, 10.0, 20.0, 30.0, 40.0, 50.0, 60.0, 70.0, 80.0, 90.0, 100.0, 110.0, 120.0, 130.0, 140.0, 150.0, 160.0, 170.0, 180.0, 190.0, 200.0, 210.0, 220.0, 230.0, 240.0, 250.0, 260.0, 270.0, 280.0, 290.0, 300.0, 310.0, 320.0, 330.0, 340.0, 350.0], "Y.HeightCorrs"=[[0.0], [-0.4], [-0.4], [-0.1], [0.6], [1.1], [1.5], [1.6], [1.5], [1.1], [0.3], [0.0], [-0.3], [-0.3], [-0.4], [0.7], [0.9], [1.8], [2.4], [2.5], [2.5], [2.2], [1.3], [0.7], [0.4], [0.0], [0.0], [0.8], [1.1], [1.7], [2.4], [2.4], [2.3], [2.3], [1.2], [0.4]], "Use Height Corrections"=FALSE}
  out "Audit Array":string[](array[string])=["Initialize", "Build TT Array", "Warm Up", "Zeroes", "AutoCal", "GlobalCalCheck", "LocalCalCheck", "Turn Table Schedule", "Vertical Corrections", "Vertical Profile", "Vertical Corrections", "Vertical Profile", "Lateral Profile", "Longitudinal Profile", "Repeat?", "Zeroes", "AutoCal", "GlobalCalCheck", "LocalCalCheck", "Turn Table Schedule", "Vertical Corrections", "Vertical Profile", "Vertical Corrections", "Vertical Profile", "Lateral Profile", "Longitudinal Profile", "Repeat?", "Zeroes", "AutoCal", "GlobalCalCheck", "LocalCalCheck", "Turn Table Schedule", "Vertical Corrections", "Vertical Profile", "Vertical Corrections", "Vertical Profile", "Lateral Profile", "Longitudinal Profile", "Repeat?", "Zeroes", "AutoCal", "GlobalCalCheck", "LocalCalCheck", "Turn Table Schedule", "Vertical Corrections", "Vertical Profile", "Vertical Corrections", "Vertical Profile", "Lateral Profile", "Longitudinal Profile", "Repeat?", "Zeroes", "AutoCal", "GlobalCalCheck", "LocalCalCheck", "Turn Table Schedule", "Vertical Corrections", "Vertical Profile", "Vertical Corrections", "Vertical Profile", "Lateral Profile", "Longitudinal Profile", "Repeat?", "Zeroes", "AutoCal", "GlobalCalCheck", "LocalCalCheck", "Turn Table Schedule", "Vertical Corrections", "Vertical Profile", "Vertical Corrections", "Vertical Profile", "Lateral Profile", "Longitudinal Profile", "Repeat?", "Zeroes", "AutoCal", "GlobalCalCheck", "LocalCalCheck", "Turn Table Schedule", "Vertical Corrections", "Vertical Profile", "Vertical Corrections", "Vertical Profile", "Lateral Profile", "Longitudinal Profile", "Repeat?", "Zeroes", "AutoCal", "GlobalCalCheck", "LocalCalCheck", "Turn Table Schedule", "Vertical Corrections", "Vertical Profile", "Vertical Corrections", "Vertical Profile", "Lateral Profile", "Longitudinal Profile", "Repeat?", "Zeroes", "AutoCal", "GlobalCalCheck", "LocalCalCheck", "Turn Table Schedule", "Vertical Corrections", "Vertical Profile", "Vertical Corrections", "Vertical Profile", "Lateral Profile", "Longitudinal Profile", "Repeat?", "Zeroes", "AutoCal", "GlobalCalCheck", "LocalCalCheck", "Turn Table Schedule", "Vertical Corrections", "Vertical Profile", "Vertical Corrections", "Vertical Profile", "Lateral Profile", "Longitudinal Profile", "Repeat?", "Zeroes", "AutoCal", "GlobalCalCheck", "LocalCalCheck", "Turn Table Schedule", "Vertical Corrections", "Vertical Profile", "Vertical Corrections", "Vertical Profile", "Lateral Profile", "Longitudinal Profile", "Repeat?", "Zeroes", "AutoCal", "GlobalCalCheck", "LocalCalCheck", "Turn Table Schedule", "Vertical Corrections", "Vertical Profile", "Vertical Corrections", "Vertical Profile", "Lateral Profile", "Longitudinal Profile", "Repeat?", "Zeroes", "AutoCal", "GlobalCalCheck", "LocalCalCheck", "Turn Table Schedule", "Vertical Corrections", "Vertical Profile", "Vertical Corrections", "Vertical Profile", "Lateral Profile", "Longitudinal Profile", "Repeat?", "Zeroes", "AutoCal", "GlobalCalCheck", "LocalCalCheck", "Turn Table Schedule", "Vertical Corrections", "Vertical Profile", "Vertical Corrections", "Vertical Profile", "Lateral Profile", "Longitudinal Profile", "Repeat?", "Zeroes", "AutoCal", "GlobalCalCheck", "LocalCalCheck", "Turn Table Schedule", "Vertical Corrections", "Vertical Profile", "Vertical Corrections", "Vertical Profile", "Lateral Profile", "Longitudinal Profile", "Repeat?", "Zeroes", "AutoCal", "GlobalCalCheck", "LocalCalCheck", "Turn Table Schedule", "Vertical Corrections", "Vertical Profile", "Vertical Corrections", "Vertical Profile", "Lateral Profile", "Longitudinal Profile", "Repeat?", "Zeroes", "AutoCal", "GlobalCalCheck", "LocalCalCheck", "Turn Table Schedule", "Vertical Corrections", "Vertical Profile", "Vertical Corrections", "Vertical Profile", "Lateral Profile", "Longitudinal Profile", "Repeat?", "Zeroes", "AutoCal", "GlobalCalCheck", "LocalCalCheck", "Turn Table Schedule", "Vertical Corrections", "Vertical Profile", "Vertical Corrections", "Vertical Profile", "Lateral Profile", "Longitudinal Profile", "Repeat?", "End"]
  in  "Index Tracking":T16
  in  "Stop Button":bool
  in  "RowTemplate":T17 {"Carrier_2 Q (l/min)" format="%#.2f"; "Row Duration (mins)" format="%#.1f"; "Row No" min=0; "Trace Gas Concentration (%)" min=0.0 format="%#_4f"; "Carrier_1 Q (l/min)" format="%#.2f"; "Tunnel Speed" format="%#.2f"; "Start X" format="%#.2f"; "Start Y" format="%#.2f"; "Start Z" format="%#.2f"; "End X" format="%#.2f"; "End Y" format="%#.2f"; "End Z" format="%#.2f"; "Averaging time (min)" min=0.0 format="%#.2f"}
  # "X           Y            Z"
  # "Start"
  # "End"
  # "X           Y            Z"
  # "Start"
  # "End"
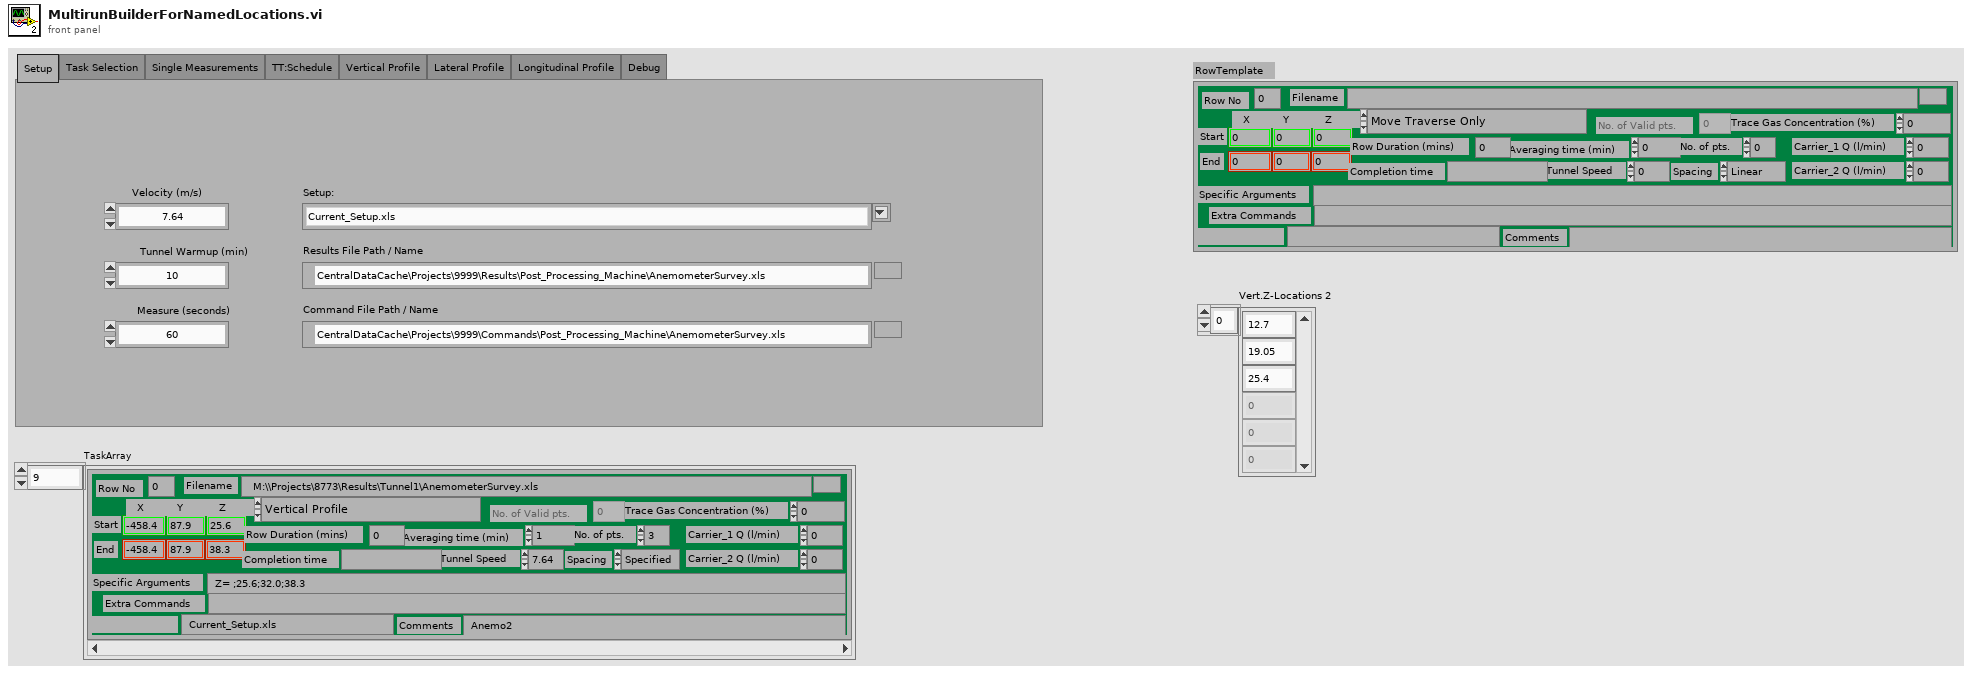
[diagram p1: front panel]
types:
  T1 = typedef "Spacing.ctl" = enum16{"Linear", "Log", "Gauss", "Specified", "N/A"}
  T2 = typedef "Multi_run_mode.ctl" = enum16{"Move Traverse Only", "Set Tunnel Speed Only", "Set Source Only", "Set Measurement Conditions", "Single Measurement", "Vertical Profile", "Lateral Profile", "Longitudinal Profile", "Explore Volume", "Multi-Axis Profile", "Auto Calibrate", "Meas Fast FID Bkgnd", "Check Beam Power", "Scanning Valve Measurement", "Run VI Named:", "Set ADAM Ch", "Wait (minutes)", "Send Message", "Synchronize With:", "Fall Back to this Row", "Turn Off Row Repeating", "Blank Row", "Traverse 3D Volume"}
  T3 = cluster{"Start X":sgl, "Start Y":sgl, "Start Z":sgl, "End X":sgl, "End Y":sgl, "End Z":sgl, "No. of pts.":i32, "Spacing":T1, "Filename":path, "Tunnel Speed":dbl, "Averaging time (min)":dbl, "Extra Commands":string, "Carrier_1 Q (l/min)":dbl, "Carrier_2 Q (l/min)":dbl, "Trace Gas Concentration (%)":dbl, "Specific Arguments":string, "Comments":string, "Row No":i32, "Row Type Selector":T2, "Completion time":string, "Row Duration (mins)":dbl, "No. of Valid pts.":i32, "Meas Setup File":string}[]
  T4 = enum32{"Setup", "Task Selection", "Single Measurements", "TT:Schedule", "Vertical Profile", "Lateral Profile", "Longitudinal Profile", "Debug"}
  T5 = cluster{"Turn Table --> Zero":bool, "AutoCal":bool, "Zeroes":bool, "Global Cal Checks":bool, "Local Cal Checks":bool, "Tunnel Off":bool}
  T6 = cluster{"Tunnel Warm Up":bool, "AutoCal":bool, "Zeroes":bool, "Turn Table Schedule":bool, "Global Cal Checks":bool, "Local Cal Checks":bool, "Vertical Profile":bool, "Lateral Profile":bool, "Reinitialize Task Array":bool, "Save Command File":bool, "Longitudinal Profile":bool}
  T7 = cluster{"X":dbl, "Y":dbl, "Z":dbl, "Use Tunnel Coords?":bool, "RepeatEveryXDeg":dbl}
  T8 = cluster{"X":dbl, "Y":dbl, "Z":dbl, "Use Tunnel Coords? Coords":bool, "RepeatEveryXDeg":dbl}
  T9 = cluster{"X":dbl, "Y":dbl, "Z":dbl, "Use Tunnel Coords?":bool, "Use Move?":bool}
  T10 = cluster{"X":dbl, "Y":dbl, "Z0":dbl, "Name":string}[]
  T11 = cluster{"TT.Azimuths":dbl[], "Z.HeightCorrs":dbl[][], "Use Height Corrections":bool, "Height Survey Filepaths":path[], "Corrections from File":bool}
  T12 = cluster{"X":dbl, "Y0":dbl, "Z":dbl, "Name":string}[]
  T13 = cluster{"Yvalues":dbl[], "X.HeightCorrs":dbl[][], "Use Height Corrections":bool}
  T14 = cluster{"X0":dbl, "Y":dbl, "Z":dbl, "Name":string}[]
  T15 = cluster{"XValues":dbl[], "Y.HeightCorrs":dbl[][], "Use Height Corrections":bool}
  T16 = cluster{"Azimuth Array Index":u32, "Vert Prof Array Index":u32, "Lat Prof Array Index":u32, "Long Prof Array Index":u32}
  T17 = cluster{"Start X":sgl, "Start Y":sgl, "Start Z":sgl, "End X":sgl, "End Y":sgl, "End Z":sgl, "No. of pts.":i32, "Spacing":T1, "Filename":path, "Tunnel Speed":dbl, "Averaging time (min)":dbl, "Extra Commands":string, "Carrier_1 Q (l/min)":dbl, "Carrier_2 Q (l/min)":dbl, "Trace Gas Concentration (%)":dbl, "Specific Arguments":string, "Comments":string, "Row No":i32, "Row Type Selector":T2, "Completion time":string, "Row Duration (mins)":dbl, "No. of Valid pts.":i32, "Meas Setup File":string}
  T18 = cluster{"Azimuth Array Index":u32, "Vert Prof Array Index":u32, "Lat Prof Array Index":u32, "Azimuth Array Index 2":u32}
  T19 = typedef "Setup_Filetype.ctl" = enum16{"Measurement Setups", "Calibration Setups", "General", "Results File Plotter Setups", "Speed Calib Tweaks"}
  T20 = cluster{"X":dbl, "Y":dbl, "Z0":dbl, "Name":string}
  T21 = cluster{"X":dbl, "Y0":dbl, "Z":dbl, "Name":string}
  T22 = cluster{"X0":dbl, "Y":dbl, "Z":dbl, "Name":string}
  T23 = enum16{"Load Command File", "Save Command File", "Check Multi Run Prog", "Check Multi Run Prog With Live Moves", "Run Multi Run Prog"}
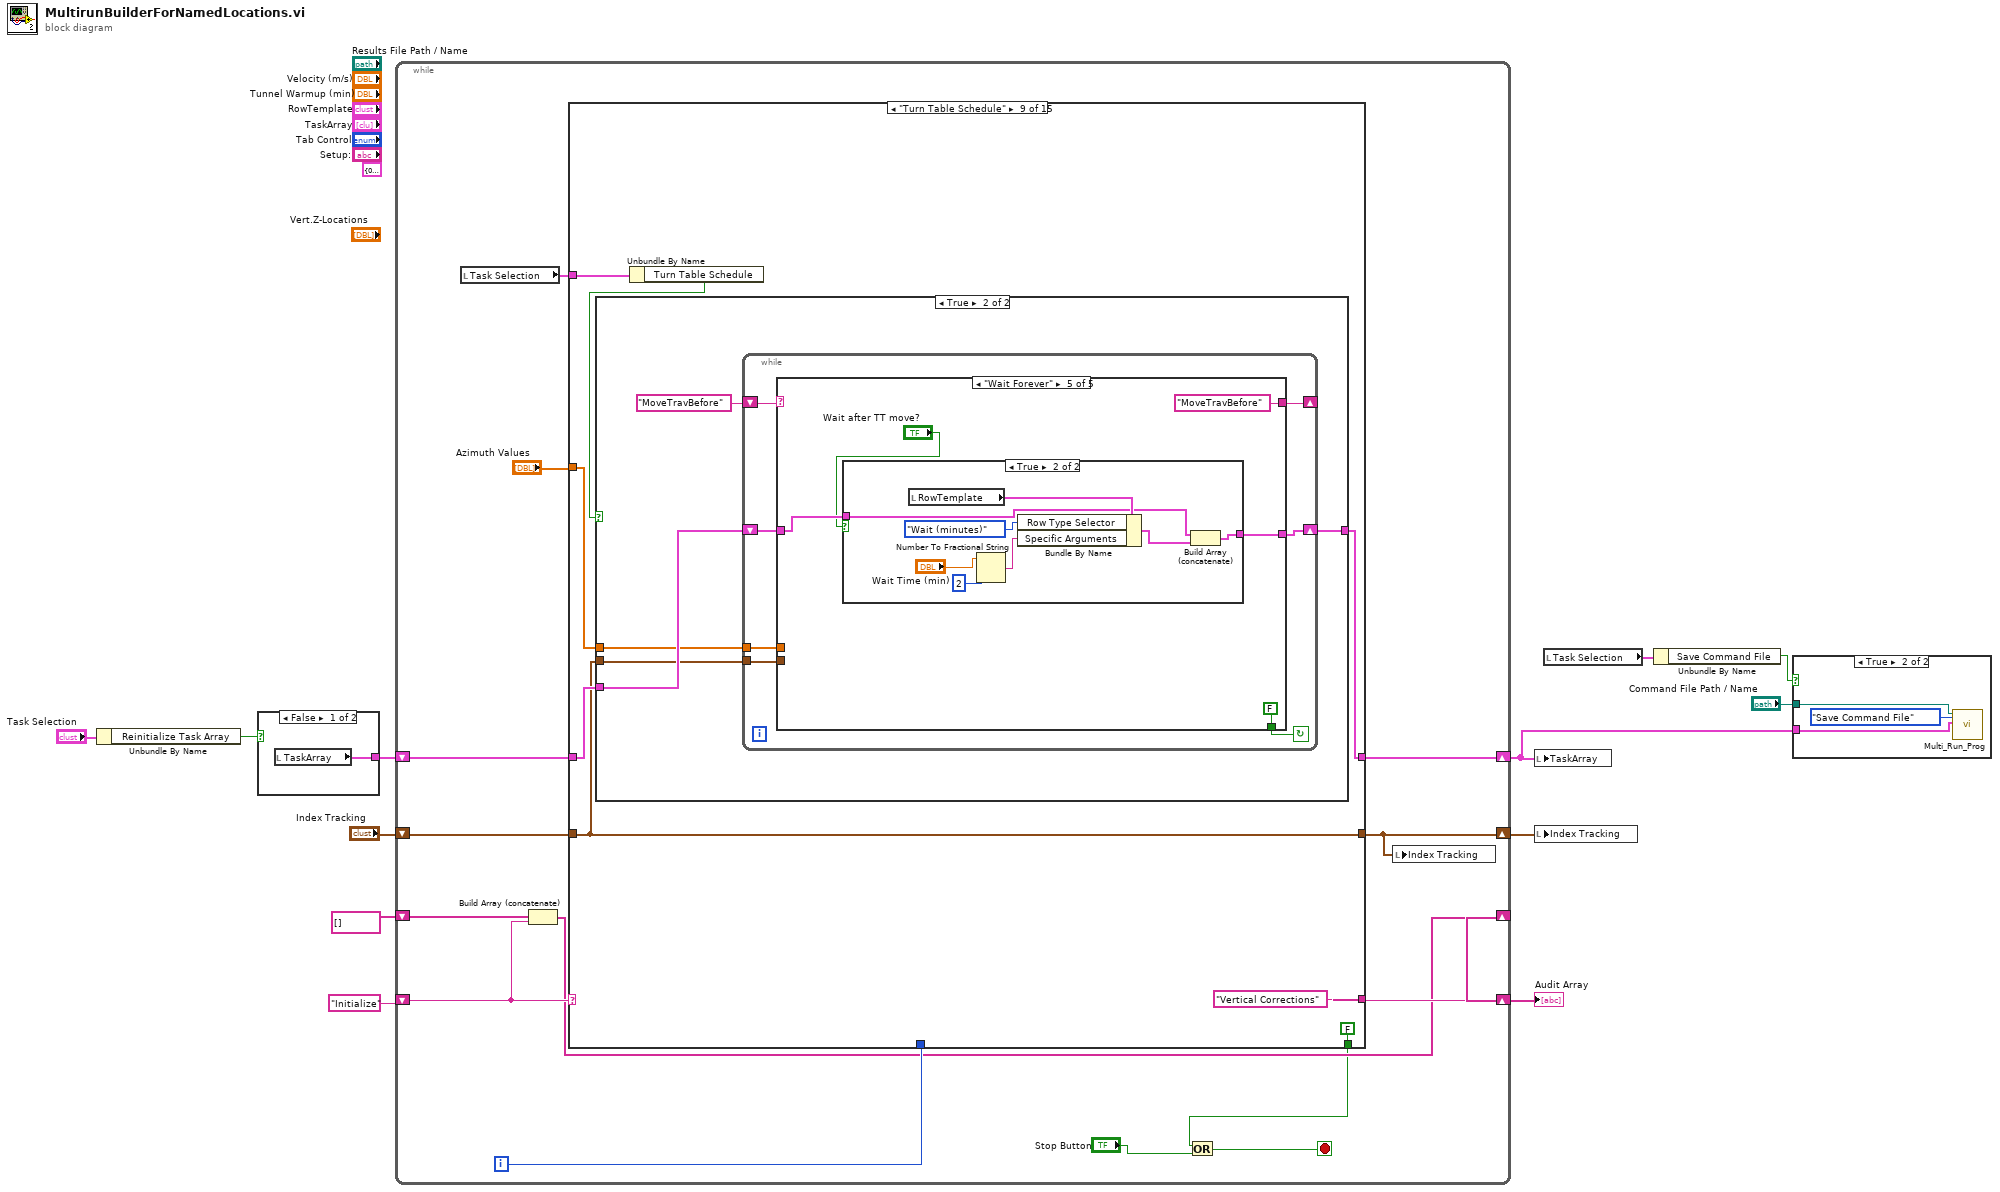
[diagram p0: block diagram]
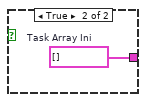
[diagram p3: hidden frame]
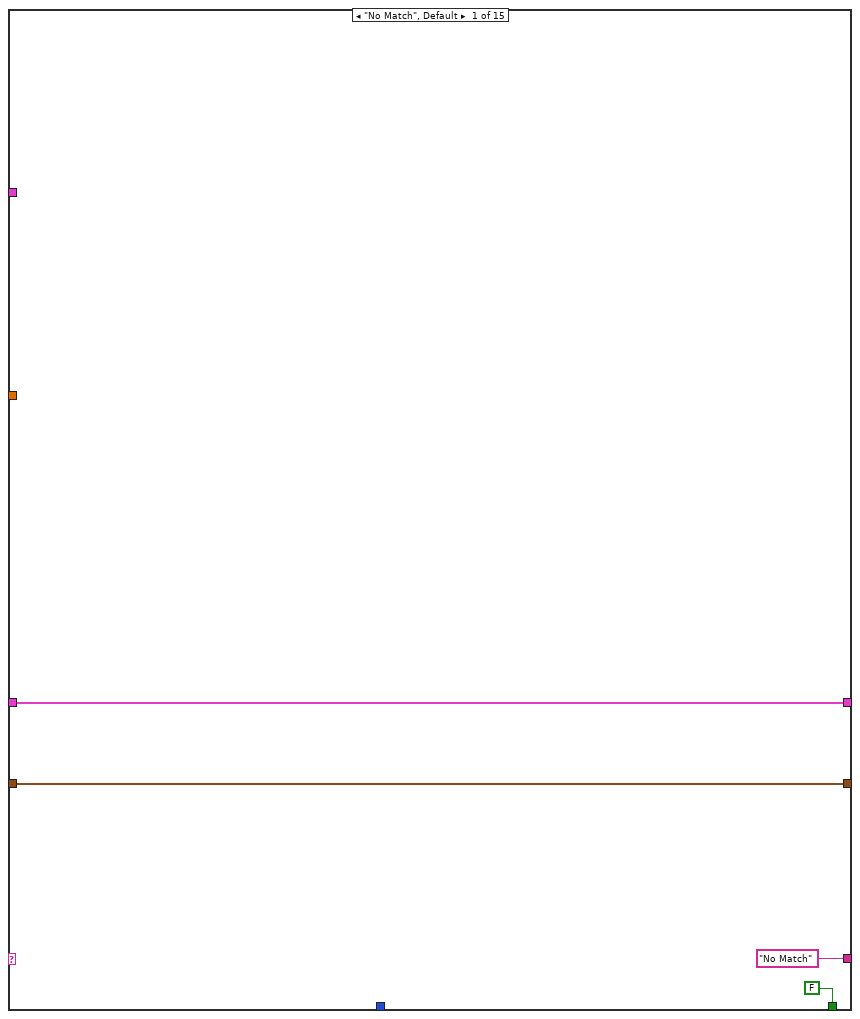
[diagram p4: hidden frame]
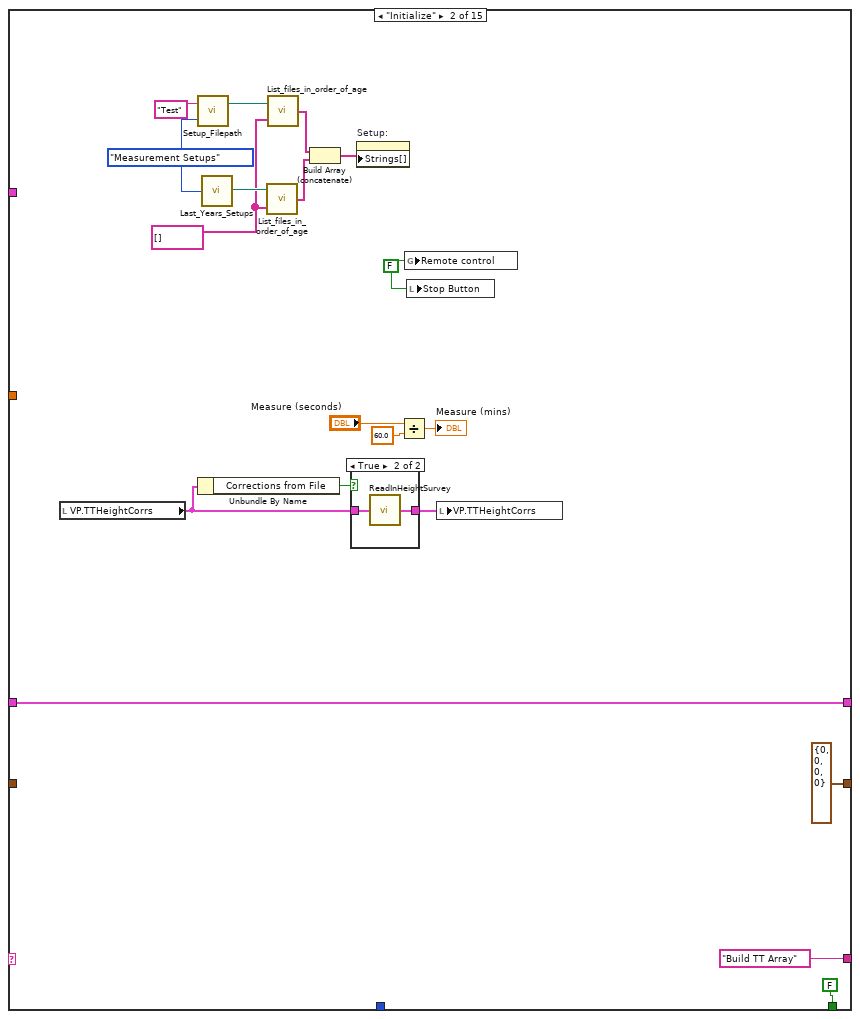
[diagram p5: hidden frame]
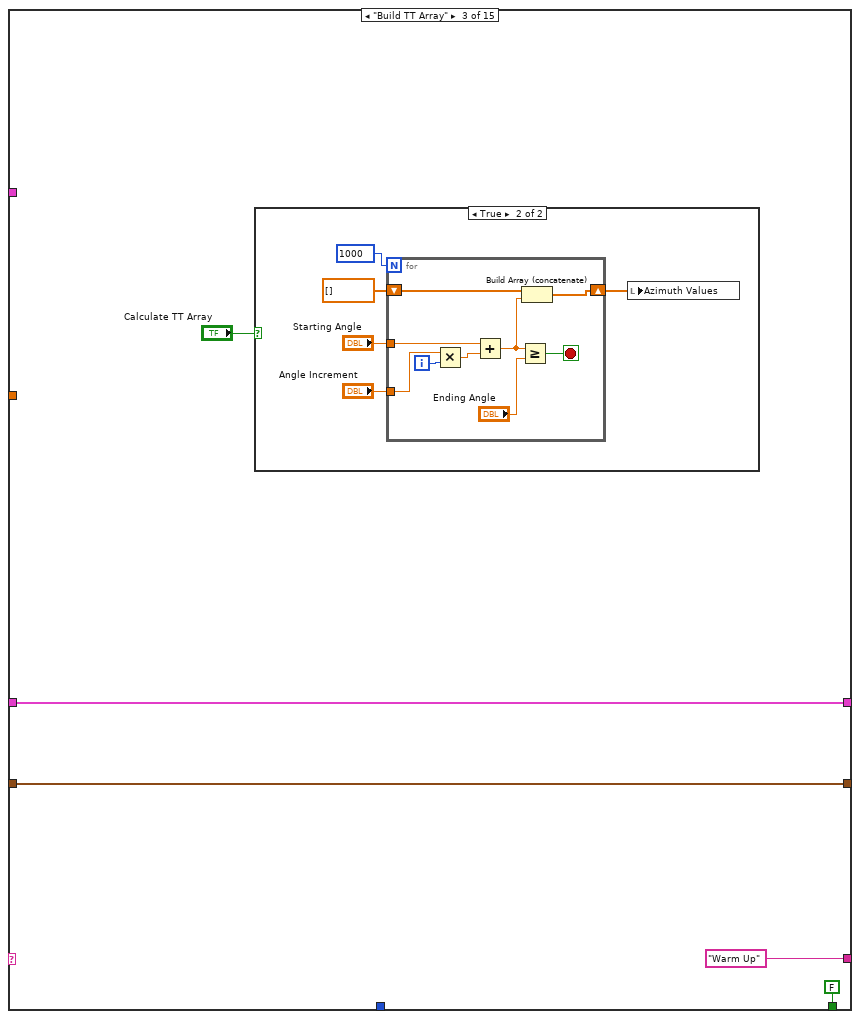
[diagram p7: hidden frame]
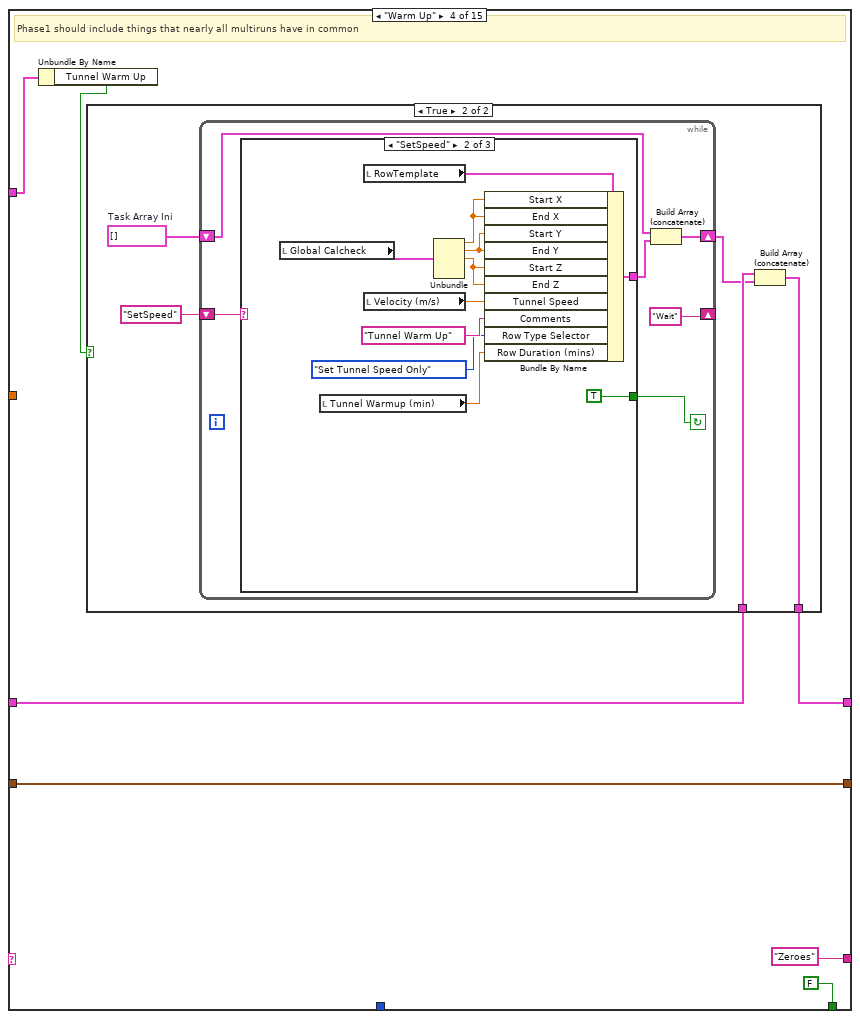
[diagram p9: hidden frame]
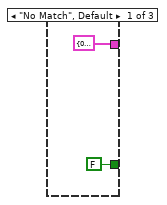
[diagram p11: hidden frame]
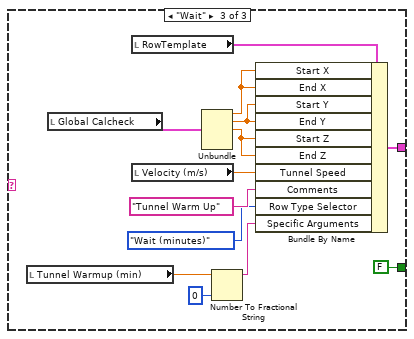
[diagram p12: hidden frame]
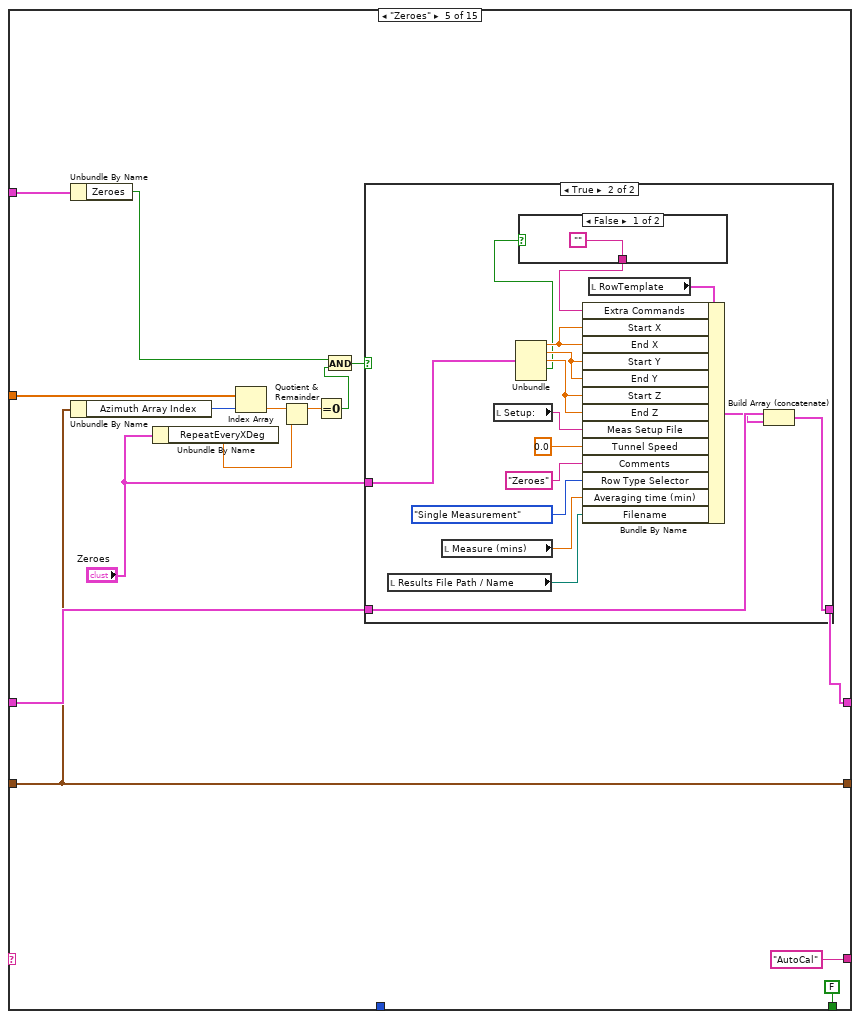
[diagram p13: hidden frame]
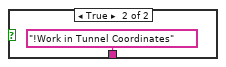
[diagram p15: hidden frame]
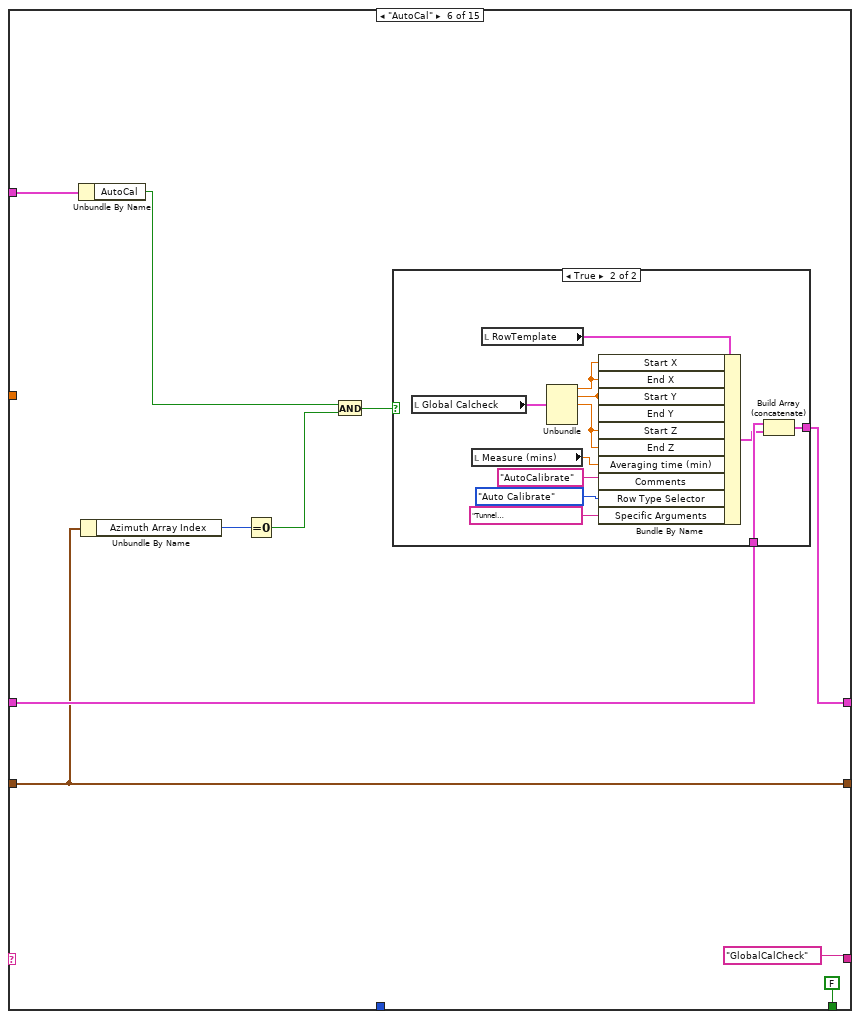
[diagram p16: hidden frame]
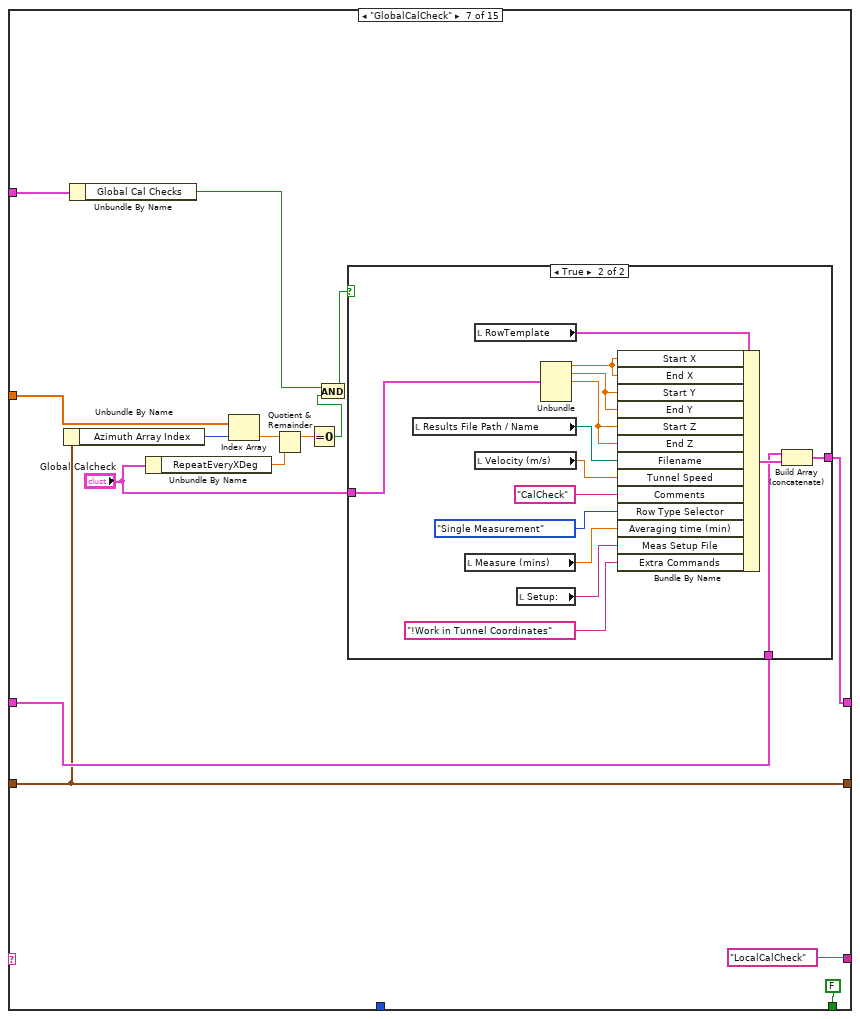
[diagram p18: hidden frame]
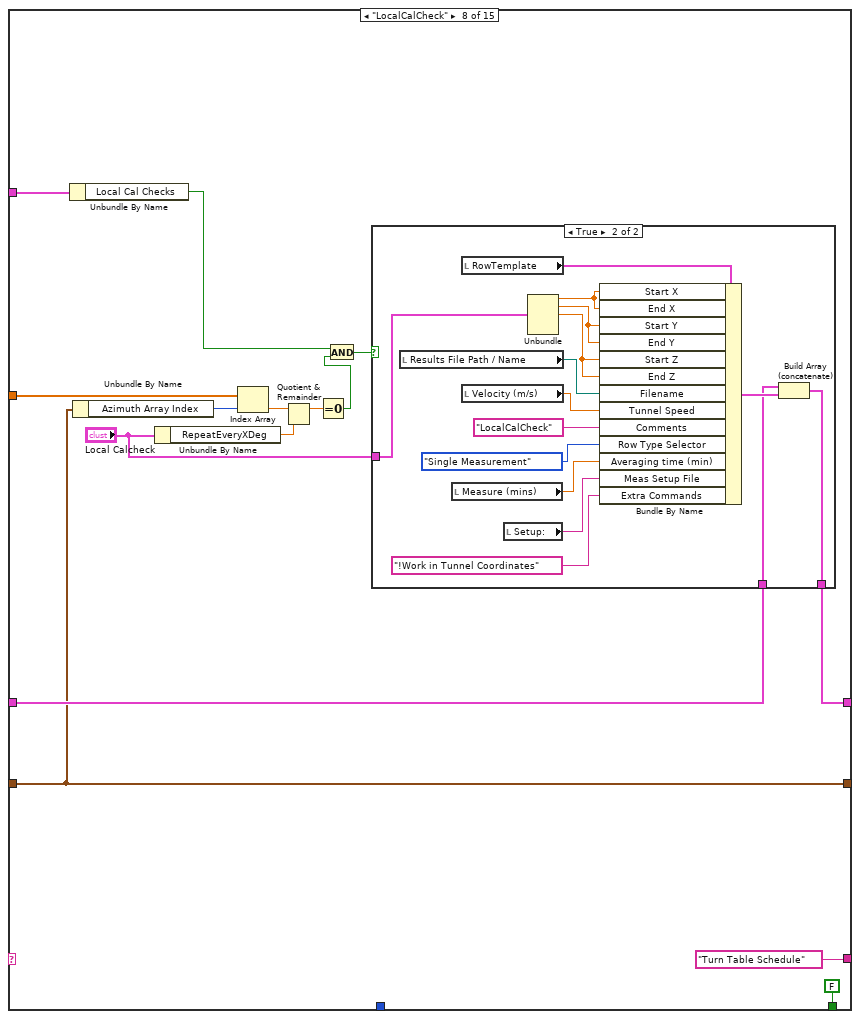
[diagram p20: hidden frame]
diagram:
  (unwired) T17 {"Start X"=0.0, "Start Y"=0.0, "Start Z"=0.0, "End X"=0.0, "End Y"=0.0, "End Z"=0.0, "No. of pts."=0, "Spacing"=enum."Linear", "Filename"=path "", "Tunnel Speed"=0.0, "Averaging time (min)"=0.0, "Extra Commands"="", "Carrier_1 Q (l/min)"=0.0, "Carrier_2 Q (l/min)"=0.0, "Trace Gas Concentration (%)"=0.0, "Specific Arguments"="", "Comments"="", "Row No"=0, "Row Type Selector"=enum."Move Traverse Only", "Completion time"="", "Row Duration (mins)"=0.0, "No. of Valid pts."=0, "Meas Setup File"=""} ("RowTemplateConst")
  n1 = Unbundle By Name("Task Selection") -> ("Reinitialize Task Array"=w9:bool)
  n2 = case shown="False" w9 {
    tunnel: [w13 w14] -> w11
    frame False {
      n3 = local read "TaskArray"() -> (w13:T3)
    }
    frame True {
      w14 = T3 []  # Task Array Ini
    }
  }
  n4 = while {
    shift-right: [w27] -> _
    shift-left: "Initialize" -> [w23]
    shift-right: [w24] -> w1
    shift-left: w11 -> [w25]
    shift-right: [w22] -> w6
    shift-left: string[] [] -> [w21]
    shift-right: [w17] -> w5
    shift-left: "Index Tracking" -> [w26]
    i -> [w28]
    stop <- w18 stop-if-true
    n5 = local read "Task Selection"() -> (w16:T6)
    n6 = Build Array (concatenate)(w21, w23) -> (w22:string[])
    n7 = case shown="\"Turn Table Schedule\"" w23 {
      tunnel: w28 -> [_ _ _ _ _ _ _ _ _ _ _ _ _ _ _]
      tunnel: ["No Match" "Build TT Array" "Warm Up" "Zeroes" "AutoCal" "GlobalCalCheck" "LocalCalCheck" "Turn Table Schedule" "Vertical Corrections" "Vertical Profile" ("t") w448 w499 w555 w606 _] -> w27
      tunnel: [FALSE ("Stop Button") FALSE ("Stop Button") FALSE ("Stop Button") FALSE ("Stop Button") FALSE ("Stop Button") FALSE ("Stop Button") FALSE ("Stop Button") FALSE ("Stop Button") FALSE ("Stop Button") FALSE FALSE ("Stop Button") FALSE ("Stop Button") FALSE ("Stop Button") FALSE ("Stop Button") TRUE] -> w19
      tunnel: "Azimuth Values" -> [_ _ _ _ w129 _ w177 w207 w242 w361 _ _ _ w605 _]
      tunnel: w26 -> [w30 _ w57 w76 w127 w157 w181 w213 w238 w363 w445 w504 w557 w611 w639]
      tunnel: [w30 T18 {"Azimuth Array Index"=0, "Vert Prof Array Index"=0, "Lat Prof Array Index"=0, "Azimuth Array Index 2"=0} ("Index Tracking") w57 w76 w127 w157 w181 w213 w238 w363 w450 w503 w556 w609 w639] -> w17
      tunnel: w25 -> [w29 w40 w58 w79 w131 w160 w188 w220 w244 w352 w452 w506 w559 w612 w635]
      tunnel: [w29 w40 w58 w78 w132 w161 w189 w221 w245 w351 w453 w507 w560 w612 w634] -> w24
      tunnel: w16 -> [_ _ _ w75 w123 w153 w180 w212 w239 _ w444 w498 w551 _ _]
      frame "No Match", Default {
      }
      frame "Initialize" {
        w36 = FALSE ("Remote control")
        w50 = Setup_Filetype."Measurement Setups" ("Setup File Type")
        w45 = string[] [] ("file names")
        n8 = local read "VP.TTHeightCorrs"() -> (w34:T11)
        n9 = call "Setup_Filepath.vi"("Setup File Type"=w50, "Filename in"="Test") -> ("Directory"=w49:path)  [unwired: 1 out]
        n10 = Unbundle By Name(w34) -> ("Corrections from File"=w35:bool)
        n11 = call "Last_Years_Setups.vi"("Setup File Type"=w50) -> ("Directory"=w51:path)
        n12 = call "List_files_in_order_of_age.vi"("Files to Hide"=w45, "Folder"=w51) -> ("file names"=w47:string[])
        n13 = call "List_files_in_order_of_age.vi"("Files to Hide"=w45, "Folder"=w49) -> ("file names"=w48:string[])
        n14 = Build Array (concatenate)(w48, w47) -> (w44:string[])
        n15 = case shown="True" w35 {
          tunnel: w34 -> [w52 w54]
          tunnel: [w52 w53] -> w33
          frame False {
          }
          frame True {
            n16 = call "ReadInHeightSurvey.vi"("VP.TTHeightCorrs In"=w54) -> ("VP.TTHeightCorrs Out"=w53:T11)
          }
        }
        n17 = property on="Setup:" class="CmbBox"("Strings[]"=w44) -> ()  [unwired: 2 in, 2 out]
        n18 = Divide(x="Measure (seconds)", y=60.0 ("x")) -> (x/y=→"Measure (mins)":dbl)
        n19 = global write "Meas_global.vi" "Remote control"(w36) -> ()
        n20 = local write "Stop Button"(w36) -> ()
        n21 = local write "VP.TTHeightCorrs"(w33) -> ()
      }
      frame "Build TT Array" {
        n22 = case shown="True" "Calculate TT Array" {
          frame False {
          }
          frame True {
            n23 = for {
              N: 1000 -> [_]
              shift-right: [w72] -> w61
              shift-left: dbl[] [] -> [w73]
              tunnel: "Starting Angle" -> [w69]
              tunnel: "Angle Increment" -> [w70]
              i -> [w71]
              stop <- w65 stop-if-true
              n24 = Multiply(x=w70, y=w71) -> (x*y=w68:dbl)
              n25 = Add(x=w69, y=w68) -> (x+y=w67:dbl)
              n26 = Greater Or Equal?(x=w67, y="Ending Angle") -> (x >= y?=w65:bool)
              n27 = Build Array (concatenate)(w73, w67) -> (w72:dbl[])
            }
            n28 = local write "Azimuth Values"(w61) -> ()
          }
        }
      }
      frame "Warm Up" {
        # "Phase1 should include things that nearly all multiruns have in common"
        n29 = Unbundle By Name(w75) -> ("Tunnel Warm Up"=w74:bool)
        n30 = case shown="True" w74 {
          tunnel: w79 -> [w81 w86]
          tunnel: [w81 w85] -> w78
          frame False {
          }
          frame True {
            w83 = T3 []  # Task Array Ini
            n31 = while {
              shift-right: ["Wait"] -> _
              shift-left: "SetSpeed" -> [w92]
              shift-right: [w89] -> w82
              shift-left: w83 -> [w88]
              stop <- w90 continue-if-true
              n32 = case shown="\"SetSpeed\"" w92 {
                tunnel: [T17 {"Start X"=0.0, "Start Y"=0.0, "Start Z"=0.0, "End X"=0.0, "End Y"=0.0, "End Z"=0.0, "No. of pts."=0, "Spacing"=enum."Linear", "Filename"=path "", "Tunnel Speed"=0.0, "Averaging time (min)"=0.0, "Extra Commands"="", "Carrier_1 Q (l/min)"=0.0, "Carrier_2 Q (l/min)"=0.0, "Trace Gas Concentration (%)"=0.0, "Specific Arguments"="", "Comments"="", "Row No"=0, "Row Type Selector"=enum."Move Traverse Only", "Completion time"="", "Row Duration (mins)"=0.0, "No. of Valid pts."=0, "Meas Setup File"=""} ("RowTemplateConst") w96 w109] -> w87
                tunnel: [FALSE TRUE FALSE] -> w90
                frame "No Match", Default {
                }
                frame "SetSpeed" {
                  n33 = local read "Global Calcheck"() -> (w100:T7)
                  n34 = local read "Tunnel Warmup (min)"() -> (w103:dbl)
                  n35 = local read "RowTemplate"() -> (w105:T17)
                  n36 = local read "Velocity (m/s)"() -> (w104:dbl)
                  n37 = Unbundle(w100) -> ("X"=w99:dbl, "Y"=w98:dbl, "Z"=w97:dbl)  [unwired: 2 out]
                  n38 = Bundle By Name(cluster=w105, "Start X"=w99, "End X"=w99, "Start Y"=w98, "End Y"=w98, "Start Z"=w97, "End Z"=w97, "Tunnel Speed"=w104, "Comments"="Tunnel Warm Up", "Row Type Selector"=Multi_run_mode."Set Tunnel Speed Only", "Row Duration (mins)"=w103) -> (w96:T17)
                }
                frame "Wait" {
                  n39 = local read "Tunnel Warmup (min)"() -> (w116:dbl)
                  n40 = local read "Global Calcheck"() -> (w113:T7)
                  n41 = local read "RowTemplate"() -> (w118:T17)
                  n42 = local read "Velocity (m/s)"() -> (w117:dbl)
                  n43 = Unbundle(w113) -> ("X"=w112:dbl, "Y"=w111:dbl, "Z"=w110:dbl)  [unwired: 2 out]
                  n44 = Number To Fractional String(number=w116, precision (6)=i16 0) -> (F-format string=w107:string)  [unwired: 2 in]
                  n45 = Bundle By Name(cluster=w118, "Start X"=w112, "End X"=w112, "Start Y"=w111, "End Y"=w111, "Start Z"=w110, "End Z"=w110, "Tunnel Speed"=w117, "Comments"="Tunnel Warm Up", "Row Type Selector"=Multi_run_mode."Wait (minutes)", "Specific Arguments"=w107) -> (w109:T17)
                }
              }
              n46 = Build Array (concatenate)(w88, w87) -> (w89:T3)
            }
            n47 = Build Array (concatenate)(w86, w82) -> (w85:T3)
          }
        }
      }
      frame "Zeroes" {
        n48 = Unbundle By Name(w123) -> ("Zeroes"=w122:bool)
        n49 = Unbundle By Name(w127) -> ("Azimuth Array Index"=w128:u32)
        n50 = Unbundle By Name("Zeroes") -> ("RepeatEveryXDeg"=w125:dbl)
        n51 = Index Array(array=w129, index=w128) -> (element=w126:dbl)
        n52 = Quotient & Remainder(x=w126, y=w125) -> (x-y*floor(x/y)=w124:dbl)  [unwired: 1 out]
        n53 = Equal To 0?(x=w124) -> (x = 0?=w121:bool)
        n54 = And(x=w122, y=w121) -> (x .and. y?=w120:bool)
        n55 = case shown="True" w120 {
          tunnel: [w134 w142] -> w132
          tunnel: w131 -> [w134 w141]
          tunnel: "Zeroes" -> [_ w135]
          frame False {
          }
          frame True {
            n56 = local read "Results File Path / Name"() -> (w138:path)
            n57 = local read "Measure (mins)"() -> (w139:dbl)
            n58 = local read "Setup:"() -> (w143:string)
            n59 = Unbundle(w135) -> ("X"=w147:dbl, "Y"=w146:dbl, "Z"=w145:dbl, "Use Tunnel Coords?"=w136:bool)  [unwired: 1 out]
            n60 = case shown="False" w136 {
              tunnel: ["" "!Work in Tunnel Coordinates"] -> w137
              frame False {
              }
              frame True {
              }
            }
            n61 = local read "RowTemplate"() -> (w150:T17)
            n62 = Bundle By Name(cluster=w150, "Extra Commands"=w137, "Start X"=w147, "End X"=w147, "Start Y"=w146, "End Y"=w146, "Start Z"=w145, "End Z"=w145, "Meas Setup File"=w143, "Tunnel Speed"=0.0, "Comments"="Zeroes", "Row Type Selector"=Multi_run_mode."Single Measurement", "Averaging time (min)"=w139, "Filename"=w138) -> (w140:T17)
            n63 = Build Array (concatenate)(w141, w140) -> (w142:T3)
          }
        }
      }
      frame "AutoCal" {
        n64 = Unbundle By Name(w153) -> ("AutoCal"=w155:bool)
        n65 = Unbundle By Name(w157) -> ("Azimuth Array Index"=w156:u32)
        n66 = Equal To 0?(x=w156) -> (x = 0?=w158:bool)
        n67 = And(x=w155, y=w158) -> (x .and. y?=w154:bool)
        n68 = case shown="True" w154 {
          tunnel: [w163 w167] -> w161
          tunnel: w160 -> [w163 w166]
          frame False {
          }
          frame True {
            n69 = local read "Global Calcheck"() -> (w172:T7)
            n70 = local read "Measure (mins)"() -> (w164:dbl)
            n71 = local read "RowTemplate"() -> (w175:T17)
            n72 = Unbundle(w172) -> ("X"=w171:dbl, "Y"=w170:dbl, "Z"=w169:dbl)  [unwired: 2 out]
            n73 = Bundle By Name(cluster=w175, "Start X"=w171, "End X"=w171, "Start Y"=w170, "End Y"=w170, "Start Z"=w169, "End Z"=w169, "Averaging time (min)"=w164, "Comments"="AutoCalibrate", "Row Type Selector"=Multi_run_mode."Auto Calibrate", "Specific Arguments"="Tunnel Speed;2.18;3.06;4.37;5.68;7.86;10.26;13.1") -> (w165:T17)
            n74 = Build Array (concatenate)(w166, w165) -> (w167:T3)
          }
        }
      }
      frame "GlobalCalCheck" {
        n75 = Unbundle By Name(w181) -> ("Azimuth Array Index"=w186:u32)
        n76 = Unbundle By Name(w180) -> ("Global Cal Checks"=w179:bool)
        n77 = Unbundle By Name("Global Calcheck") -> ("RepeatEveryXDeg"=w184:dbl)
        n78 = Index Array(array=w177, index=w186) -> (element=w185:dbl)
        n79 = Quotient & Remainder(x=w185, y=w184) -> (x-y*floor(x/y)=w183:dbl)  [unwired: 1 out]
        n80 = Equal To 0?(x=w183) -> (x = 0?=w182:bool)
        n81 = And(x=w179, y=w182) -> (x .and. y?=w176:bool)
        n82 = case shown="True" w176 {
          tunnel: [w191 w196] -> w189
          tunnel: w188 -> [w191 w194]
          tunnel: "Global Calcheck" -> [_ w192]
          frame False {
          }
          frame True {
            n83 = local read "Results File Path / Name"() -> (w198:path)
            n84 = local read "Measure (mins)"() -> (w204:dbl)
            n85 = local read "RowTemplate"() -> (w206:T17)
            n86 = local read "Velocity (m/s)"() -> (w205:dbl)
            n87 = local read "Setup:"() -> (w197:string)
            n88 = Unbundle(w192) -> ("X"=w201:dbl, "Y"=w200:dbl, "Z"=w199:dbl)  [unwired: 2 out]
            n89 = Bundle By Name(cluster=w206, "Start X"=w201, "End X"=w201, "Start Y"=w200, "End Y"=w200, "Start Z"=w199, "End Z"=w199, "Filename"=w198, "Tunnel Speed"=w205, "Comments"="CalCheck", "Row Type Selector"=Multi_run_mode."Single Measurement", "Averaging time (min)"=w204, "Meas Setup File"=w197, "Extra Commands"="!Work in Tunnel Coordinates") -> (w195:T17)
            n90 = Build Array (concatenate)(w194, w195) -> (w196:T3)
          }
        }
      }
      frame "LocalCalCheck" {
        n91 = Unbundle By Name(w212) -> ("Local Cal Checks"=w211:bool)
        n92 = Unbundle By Name(w213) -> ("Azimuth Array Index"=w217:u32)
        n93 = Unbundle By Name("Local Calcheck") -> ("RepeatEveryXDeg"=w215:dbl)
        n94 = Index Array(array=w207, index=w217) -> (element=w216:dbl)
        n95 = Quotient & Remainder(x=w216, y=w215) -> (x-y*floor(x/y)=w214:dbl)  [unwired: 1 out]
        n96 = Equal To 0?(x=w214) -> (x = 0?=w210:bool)
        n97 = And(x=w211, y=w210) -> (x .and. y?=w209:bool)
        n98 = case shown="True" w209 {
          tunnel: [w222 w227] -> w221
          tunnel: w220 -> [w222 w225]
          tunnel: "Local Calcheck" -> [_ w223]
          frame False {
          }
          frame True {
            n99 = local read "Results File Path / Name"() -> (w229:path)
            n100 = local read "Measure (mins)"() -> (w228:dbl)
            n101 = local read "RowTemplate"() -> (w237:T17)
            n102 = local read "Velocity (m/s)"() -> (w236:dbl)
            n103 = local read "Setup:"() -> (w230:string)
            n104 = Unbundle(w223) -> ("X"=w233:dbl, "Y"=w232:dbl, "Z"=w231:dbl)  [unwired: 2 out]
            n105 = Bundle By Name(cluster=w237, "Start X"=w233, "End X"=w233, "Start Y"=w232, "End Y"=w232, "Start Z"=w231, "End Z"=w231, "Filename"=w229, "Tunnel Speed"=w236, "Comments"="LocalCalCheck", "Row Type Selector"=Multi_run_mode."Single Measurement", "Averaging time (min)"=w228, "Meas Setup File"=w230, "Extra Commands"="!Work in Tunnel Coordinates") -> (w226:T17)
            n106 = Build Array (concatenate)(w225, w226) -> (w227:T3)
          }
        }
      }
      frame "Turn Table Schedule" {
        n107 = Unbundle By Name(w239) -> ("Turn Table Schedule"=w240:bool)
        n108 = case shown="True" w240 {
          tunnel: [w246 w251] -> w245
          tunnel: w244 -> [w246 w250]
          tunnel: w242 -> [_ w249]
          tunnel: w238 -> [_ w248]
          frame False {
          }
          frame True {
            n109 = while {
              tunnel: w249 -> [w258]
              tunnel: w248 -> [w257]
              shift-right: [w254] -> w251
              shift-left: w250 -> [w255]
              shift-right: [w252] -> _
              shift-left: "MoveTravBefore" -> [w256]
              stop <- w253 continue-if-true
              n110 = case shown="\"Wait Forever\"" w256 {
                tunnel: [w262 w283 w307 w328 w340] -> w254
                tunnel: w258 -> [_ w289 _ _ _]
                tunnel: w257 -> [_ w286 _ _ _]
                tunnel: w255 -> [w263 w282 w308 w327 w339]
                tunnel: [TRUE TRUE TRUE TRUE FALSE] -> w253
                tunnel: ["MoveTT" "MoveTravAfter" "Send Message" "Wait Forever" "MoveTravBefore"] -> w252
                frame "MoveTravBefore" {
                  n111 = Unbundle By Name("MoveTravBeforeTT") -> ("Use Move?"=w264:bool)
                  n112 = case shown="False" w264 {
                    tunnel: "MoveTravBeforeTT" -> [_ w269]
                    tunnel: w263 -> [w265 w268]
                    tunnel: [w265 w266] -> w262
                    frame False {
                    }
                    frame True {
                      n113 = local read "Velocity (m/s)"() -> (w276:dbl)
                      n114 = Unbundle(w269) -> ("X"=w274:dbl, "Y"=w273:dbl, "Z"=w272:dbl, "Use Tunnel Coords?"=w271:bool)  [unwired: 1 out]
                      n115 = case shown="False" w271 {
                        tunnel: ["" "!Work in Tunnel Coordinates"] -> w270
                        frame False {
                        }
                        frame True {
                        }
                      }
                      n116 = local read "RowTemplate"() -> (w277:T17)
                      n117 = Bundle By Name(cluster=w277, "Extra Commands"=w270, "Start X"=w274, "End X"=w274, "Start Y"=w273, "End Y"=w273, "Start Z"=w272, "End Z"=w272, "Tunnel Speed"=w276, "Row Type Selector"=Multi_run_mode."Move Traverse Only") -> (w267:T17)
                      n118 = Build Array (concatenate)(w268, w267) -> (w266:T3)
                    }
                  }
                }
                frame "MoveTT", Default {
                  n119 = Unbundle By Name(w286) -> ("Azimuth Array Index"=w285:u32)
                  n120 = local read "Local Calcheck"() -> (w298:T8)
                  n121 = Index Array(array=w289, index=w285) -> (element=w292:dbl)
                  n122 = local read "Velocity (m/s)"() -> (w300:dbl)
                  n123 = Number To Fractional String(number=w292, precision (6)=i16 0) -> (F-format string=w291:string)  [unwired: 2 in]
                  n124 = Unbundle(w298) -> ("X"=w297:dbl, "Y"=w296:dbl, "Z"=w295:dbl, "Use Tunnel Coords? Coords"=w288:bool)  [unwired: 1 out]
                  n125 = case shown="False" w288 {
                    tunnel: ["" "!Work in Tunnel Coordinates"] -> w287
                    frame False {
                    }
                    frame True {
                    }
                  }
                  n126 = Concatenate Strings("MoveTT.vi;" ("Specific Arguments"), w291) -> (w293:string)
                  n127 = local read "RowTemplate"() -> (w301:T17)
                  n128 = Bundle By Name(cluster=w301, "Extra Commands"=w287, "Start X"=w297, "End X"=w297, "Start Y"=w296, "End Y"=w296, "Start Z"=w295, "End Z"=w295, "Tunnel Speed"=w300, "Row Type Selector"=Multi_run_mode."Run VI Named:", "Specific Arguments"=w293) -> (w284:T17)
                  n129 = Build Array (concatenate)(w282, w284) -> (w283:T3)
                }
                frame "MoveTravAfter" {
                  n130 = Unbundle By Name("MoveTravAfterTT") -> ("Use Move?"=w309:bool)
                  n131 = case shown="True" w309 {
                    tunnel: "MoveTravAfterTT" -> [_ w314]
                    tunnel: w308 -> [w310 w311]
                    tunnel: [w310 w313] -> w307
                    frame False {
                    }
                    frame True {
                      n132 = local read "Velocity (m/s)"() -> (w321:dbl)
                      n133 = Unbundle(w314) -> ("X"=w319:dbl, "Y"=w318:dbl, "Z"=w317:dbl, "Use Tunnel Coords?"=w316:bool)  [unwired: 1 out]
                      n134 = case shown="False" w316 {
                        tunnel: ["" "!Work in Tunnel Coordinates"] -> w315
                        frame False {
                        }
                        frame True {
                        }
                      }
                      n135 = local read "RowTemplate"() -> (w322:T17)
                      n136 = Bundle By Name(cluster=w322, "Extra Commands"=w315, "Start X"=w319, "End X"=w319, "Start Y"=w318, "End Y"=w318, "Start Z"=w317, "End Z"=w317, "Tunnel Speed"=w321, "Row Type Selector"=Multi_run_mode."Move Traverse Only") -> (w312:T17)
                      n137 = Build Array (concatenate)(w311, w312) -> (w313:T3)
                    }
                  }
                }
                frame "Send Message" {
                  n138 = case shown="True" "Send Message after TT move?" {
                    tunnel: [w330 w332] -> w328
                    tunnel: w327 -> [w330 w331]
                    frame False {
                    }
                    frame True {
                      n139 = local read "RowTemplate"() -> (w336:T17)
                      n140 = Bundle By Name(cluster=w336, "Row Type Selector"=Multi_run_mode."Send Message", "Comments"="Message") -> (w333:T17)
                      n141 = Build Array (concatenate)(w331, w333) -> (w332:T3)
                    }
                  }
                }
                frame "Wait Forever" {
                  n142 = case shown="True" "Wait after TT move?" {
                    tunnel: [w342 w345] -> w340
                    tunnel: w339 -> [w342 w344]
                    frame False {
                    }
                    frame True {
                      n143 = local read "RowTemplate"() -> (w350:T17)
                      n144 = Number To Fractional String(number="Wait Time (min)", precision (6)=i16 2) -> (F-format string=w347:string)  [unwired: 2 in]
                      n145 = Bundle By Name(cluster=w350, "Row Type Selector"=Multi_run_mode."Wait (minutes)", "Specific Arguments"=w347) -> (w346:T17)
                      n146 = Build Array (concatenate)(w344, w346) -> (w345:T3)
                    }
                  }
                }
              }
            }
          }
        }
      }
      frame "Vertical Corrections" {
        # "In order to actually use height corrections for Lateral & Longitudinal Profiles, a Multi-axis Profile should be used instead..."
        n147 = Unbundle By Name(w363) -> ("Azimuth Array Index"=w362:u32, "Vert Prof Array Index"=w356:u32, "Lat Prof Array Index"=w357:u32, "Long Prof Array Index"=w358:u32)
        n148 = Index Array(array=w361, index=w362) -> (element=w360:dbl)
        n149 = while {
          tunnel: w360 -> [w377]
          shift-right: [w375] -> _
          shift-left: "Vertical" -> [w376]
          tunnel: w358 -> [w371]
          tunnel: w357 -> [w372]
          tunnel: w356 -> [w373]
          tunnel: "VP.TTHeightCorrs" -> [w370]
          tunnel: "Lat.HeightCorrs" -> [w369]
          tunnel: "Long.HeightCorrs" -> [w368]
          tunnel: w352 -> [w367]
          tunnel: [w366] -> w351
          stop <- w374 continue-if-true
          n150 = case shown="\"Vertical\", Default" w376 {
            tunnel: w377 -> [_ w387 w411 w429]
            tunnel: [_ "Lateral" "Longitudinal" _] -> w375
            tunnel: [FALSE FALSE TRUE FALSE] -> w374
            tunnel: w373 -> [_ w384 _ _]
            tunnel: w372 -> [_ _ w407 _]
            tunnel: w371 -> [_ _ _ w426]
            tunnel: w370 -> [_ w382 _ _]
            tunnel: w369 -> [_ _ w408 _]
            tunnel: w368 -> [_ _ _ w427]
            tunnel: w367 -> [w378 w381 w406 w425]
            tunnel: [w378 w380 w406 w425] -> w366
            frame "No Match" {
            }
            frame "Vertical", Default {
              n151 = Unbundle By Name(w382) -> ("Use Height Corrections"=w383:bool)
              n152 = case shown="True" w383 {
                tunnel: w387 -> [_ w404]
                tunnel: w384 -> [_ w399]
                tunnel: w382 -> [_ w398]
                tunnel: w381 -> [w388 w390]
                tunnel: [w388 w389] -> w380
                frame False {
                }
                frame True {
                  n153 = Unbundle By Name(w398) -> ("TT.Azimuths"=w405:dbl[], "Z.HeightCorrs"=w403:dbl[][])
                  n154 = local read "Vert.Z-Locations"() -> (w402:dbl[])
                  n155 = Search 1D Array(1D array=w405, element=w404) -> (index of element=w400:i32)  [unwired: 1 in]
                  n156 = Index Array(array=w403, index (row)=w400, index (col)=w399) -> (element=w394:dbl)
                  n157 = Number To Fractional String(number=w394, precision (6)=i16 3) -> (F-format string=w392:string)  [unwired: 2 in]
                  n158 = Add(x=w402, y=w394) -> (x+y=w401:dbl[])
                  n159 = local read "RowTemplate"() -> (w395:T17)
                  n160 = Bundle By Name(cluster=w395, "Row Type Selector"=Multi_run_mode."Set ADAM Ch", "Specific Arguments"="Correction Channel Name", "Extra Commands"=w392) -> (w391:T17)
                  n161 = local write "Vert.Z-Locations 2"(w401) -> ()
                  n162 = Build Array (concatenate)(w390, w391) -> (w389:T3)
                }
              }
            }
            frame "Lateral" {
              n163 = disable-structure shown="Disabled" {
                disable-tunnel: w411 -> [w415 _]
                disable-tunnel: w408 -> [w413 _]
                disable-tunnel: w407 -> [w412 _]
                frame Disabled {
                  n164 = Unbundle By Name(w413) -> ("Use Height Corrections"=w414:bool)
                  n165 = case shown="True" w414 {
                    tunnel: w415 -> [_ w423]
                    tunnel: w412 -> [_ w417]
                    tunnel: w413 -> [_ w416]
                    frame False {
                    }
                    frame True {
                      n166 = Unbundle By Name(w416) -> ("Yvalues"=w424:dbl[], "X.HeightCorrs"=w422:dbl[][])
                      n167 = local read "Vert.Z-Locations"() -> (w421:dbl[])
                      n168 = Search 1D Array(1D array=w424, element=w423) -> (index of element=w418:i32)  [unwired: 1 in]
                      n169 = Index Array(array=w422, index (row)=w418, index (col)=w417) -> (element=w420:dbl)
                      n170 = Add(x=w421, y=w420) -> (x+y=w419:dbl[])
                      n171 = local write "Vert.Z-Locations 2"(w419) -> ()
                    }
                  }
                }
                frame Enabled {
                }
              }
            }
            frame "Longitudinal" {
              n172 = disable-structure shown="Disabled" {
                disable-tunnel: w429 -> [w433 _]
                disable-tunnel: w427 -> [w431 _]
                disable-tunnel: w426 -> [w430 _]
                frame Disabled {
                  n173 = Unbundle By Name(w431) -> ("Use Height Corrections"=w432:bool)
                  n174 = case shown="True" w432 {
                    tunnel: w433 -> [_ w441]
                    tunnel: w430 -> [_ w435]
                    tunnel: w431 -> [_ w434]
                    frame False {
                    }
                    frame True {
                      n175 = Unbundle By Name(w434) -> ("XValues"=w442:dbl[], "Y.HeightCorrs"=w440:dbl[][])
                      n176 = local read "Vert.Z-Locations"() -> (w439:dbl[])
                      n177 = Search 1D Array(1D array=w442, element=w441) -> (index of element=w436:i32)  [unwired: 1 in]
                      n178 = Index Array(array=w440, index (row)=w436, index (col)=w435) -> (element=w438:dbl)
                      n179 = Add(x=w439, y=w438) -> (x+y=w437:dbl[])
                      n180 = local write "Vert.Z-Locations 2"(w437) -> ()
                    }
                  }
                }
                frame Enabled {
                }
              }
            }
          }
        }
      }
      frame "Vertical Profile" {
        n181 = Unbundle By Name(w444) -> ("Vertical Profile"=w443:bool)
        n182 = case shown="True" w443 {
          tunnel: [w456 w484] -> w453
          tunnel: w452 -> [w456 w482]
          tunnel: [w455 w481] -> w450
          tunnel: [TRUE w476] -> w446
          tunnel: w445 -> [w455 w475]
          frame False {
          }
          frame True {
            n183 = Array Size(array="Vert.Z-Locations 2") -> (size(s)=w462:i32)
            n184 = local read "Results File Path / Name"() -> (w469:path)
            n185 = Array Size(array="VertProf.Coords") -> (size(s)=w477:i32)
            n186 = Decrement(x=w462) -> (x-1=w485:i32)
            n187 = Decrement(x=w477) -> (x-1=w458:i32)
            n188 = in-place {
              in-place-border: [w491] -> w480
              in-place-border: w458 -> [w490]
              in-place-border: [w492] -> w476
              n189 = in-place-cluster #1(w475) -> ("Vert Prof Array Index"=w491:u32)
              n190 = Equal?(x=w490, y=w491) -> (x = y?=w492:bool)
              n191 = case shown="False" w492 {
                tunnel: [w494 u32 0] -> w493
                tunnel: w491 -> [w495 _]
                frame False {
                  n192 = Increment(x=w495) -> (x+1=w494:u32)
                }
                frame True {
                }
              }
              n193 = in-place-cluster #1("Vert Prof Array Index"=w493) -> (w481:T16)
            }
            n194 = Index Array(array="VertProf.Coords", index=w480) -> (element=w488:T20)
            n195 = Unbundle By Name(w488) -> ("Z0"=w466:dbl, "X"=w461:dbl, "Y"=w460:dbl, "Name"=w459:string)
            n196 = Add(x=w466, y="Vert.Z-Locations 2") -> (x+y=w467:dbl[])
            n197 = Array To Spreadsheet String(delimiter (Tab)=";", array=w467, 3:"%.1f" ("format string")) -> (spreadsheet string=w479:string)
            n198 = Index Array(array=w467, index #2=w485) -> (element #1=w464:dbl, element #2=w463:dbl)  [unwired: 1 in]
            n199 = local read "Measure (mins)"() -> (w470:dbl)
            n200 = local read "Velocity (m/s)"() -> (w471:dbl)
            n201 = local read "Setup:"() -> (w468:string)
            n202 = Concatenate Strings("Z= ;", w479) -> (w465:string)
            n203 = local read "RowTemplate"() -> (w489:T17)
            n204 = Bundle By Name(cluster=w489, "Row Type Selector"=Multi_run_mode."Vertical Profile", "Spacing"=Spacing."Specified", "Tunnel Speed"=w471, "Averaging time (min)"=w470, "Filename"=w469, "Meas Setup File"=w468, "Specific Arguments"=w465, "Start Z"=w464, "End Z"=w463, "No. of pts."=w462, "Start X"=w461, "End X"=w461, "Start Y"=w460, "End Y"=w460, "Comments"=w459) -> (w483:T17)
            n205 = Build Array (concatenate)(w482, w483) -> (w484:T3)
          }
        }
        n206 = Select(t="Lateral Profile", s=w446, f="Vertical Corrections") -> (s? t:f=w448:string)
      }
      frame "Lateral Profile" {
        n207 = Unbundle By Name(w498) -> ("Lateral Profile"=w497:bool)
        n208 = case shown="False" w497 {
          tunnel: [w508 w541] -> w507
          tunnel: w506 -> [w508 w540]
          tunnel: w504 -> [w509 w539]
          tunnel: [w509 w538] -> w503
          tunnel: [TRUE w534] -> w500
          frame False {
          }
          frame True {
            n209 = Array Size(array="Lat.Y-Locations") -> (size(s)=w515:i32)
            n210 = local read "Results File Path / Name"() -> (w527:path)
            n211 = Decrement(x=w515) -> (x-1=w522:i32)
            n212 = Array To Spreadsheet String(delimiter (Tab)=";", array="Lat.Y-Locations", 3:"%.1f" ("format string")) -> (spreadsheet string=w521:string)
            n213 = local read "Measure (mins)"() -> (w528:dbl)
            n214 = Array Size(array="LatProf.Coords") -> (size(s)=w536:i32)
            n215 = Index Array(array="Lat.Y-Locations", index #1=0 ("index"), index #2=w522) -> (element #1=w517:dbl, element #2=w516:dbl)
            n216 = local read "Velocity (m/s)"() -> (w529:dbl)
            n217 = Decrement(x=w536) -> (x-1=w535:i32)
            n218 = in-place {
              in-place-border: [w544] -> w537
              in-place-border: w535 -> [w545]
              in-place-border: [w543] -> w534
              n219 = in-place-cluster #2(w539) -> ("Lat Prof Array Index"=w544:u32)
              n220 = Equal?(x=w545, y=w544) -> (x = y?=w543:bool)
              n221 = case shown="True" w543 {
                tunnel: [w548 u32 0] -> w546
                tunnel: w544 -> [w547 _]
                frame False {
                  n222 = Increment(x=w547) -> (x+1=w548:u32)
                }
                frame True {
                }
              }
              n223 = in-place-cluster #2("Lat Prof Array Index"=w546) -> (w538:T16)
            }
            n224 = Index Array(array="LatProf.Coords", index=w537) -> (element=w542:T21)
            n225 = Unbundle By Name(w542) -> ("X"=w514:dbl, "Z"=w513:dbl, "Name"=w512:string)
            n226 = local read "Setup:"() -> (w526:string)
            n227 = Concatenate Strings("Y= ;", w521) -> (w518:string)
            n228 = local read "RowTemplate"() -> (w532:T17)
            n229 = Bundle By Name(cluster=w532, "Row Type Selector"=Multi_run_mode."Lateral Profile", "Spacing"=Spacing."Specified", "Tunnel Speed"=w529, "Averaging time (min)"=w528, "Filename"=w527, "Meas Setup File"=w526, "Specific Arguments"=w518, "Start Y"=w517, "End Y"=w516, "No. of pts."=w515, "Start X"=w514, "End X"=w514, "Start Z"=w513, "End Z"=w513, "Comments"=w512) -> (w511:T17)
            n230 = Build Array (concatenate)(w540, w511) -> (w541:T3)
          }
        }
        n231 = Select(t="Longitudinal Profile", s=w500, f="Lateral Profile") -> (s? t:f=w499:string)
      }
      frame "Longitudinal Profile" {
        n232 = Unbundle By Name(w551) -> ("Longitudinal Profile"=w550:bool)
        n233 = case shown="True" w550 {
          tunnel: [w563 w593] -> w560
          tunnel: w559 -> [w563 w591]
          tunnel: w557 -> [w562 w590]
          tunnel: [w562 w589] -> w556
          tunnel: [TRUE w584] -> w554
          frame False {
          }
          frame True {
            n234 = Array Size(array="Long.X-Locations") -> (size(s)=w567:i32)
            n235 = local read "Results File Path / Name"() -> (w579:path)
            n236 = Decrement(x=w567) -> (x-1=w574:i32)
            n237 = Array To Spreadsheet String(delimiter (Tab)=";", array="Long.X-Locations", 3:"%.1f" ("format string")) -> (spreadsheet string=w573:string)
            n238 = local read "Measure (mins)"() -> (w580:dbl)
            n239 = Array Size(array="LongProf.Coords") -> (size(s)=w587:i32)
            n240 = local read "Velocity (m/s)"() -> (w581:dbl)
            n241 = Index Array(array="Long.X-Locations", index #1=0 ("index"), index #2=w574) -> (element #1=w569:dbl, element #2=w568:dbl)
            n242 = Decrement(x=w587) -> (x-1=w585:i32)
            n243 = in-place {
              in-place-border: [w598] -> w588
              in-place-border: w585 -> [w597]
              in-place-border: [w596] -> w584
              n244 = in-place-cluster #3(w590) -> ("Long Prof Array Index"=w598:u32)
              n245 = Equal?(x=w597, y=w598) -> (x = y?=w596:bool)
              n246 = case shown="True" w596 {
                tunnel: [w601 u32 0] -> w599
                tunnel: w598 -> [w600 _]
                frame False {
                  n247 = Increment(x=w600) -> (x+1=w601:u32)
                }
                frame True {
                }
              }
              n248 = in-place-cluster #3("Long Prof Array Index"=w599) -> (w589:T16)
            }
            n249 = Index Array(array="LongProf.Coords", index=w588) -> (element=w594:T22)
            n250 = Unbundle By Name(w594) -> ("Y"=w566:dbl, "Z"=w565:dbl, "Name"=w564:string)
            n251 = local read "Setup:"() -> (w578:string)
            n252 = Concatenate Strings("X= ;", w573) -> (w570:string)
            n253 = local read "RowTemplate"() -> (w595:T17)
            n254 = Bundle By Name(cluster=w595, "Row Type Selector"=Multi_run_mode."Longitudinal Profile", "Spacing"=Spacing."Specified", "Tunnel Speed"=w581, "Averaging time (min)"=w580, "Filename"=w579, "Meas Setup File"=w578, "Specific Arguments"=w570, "Start X"=w569, "End X"=w568, "No. of pts."=w567, "Start Y"=w566, "End Y"=w566, "Start Z"=w565, "End Z"=w565, "Comments"=w564) -> (w592:T17)
            n255 = Build Array (concatenate)(w591, w592) -> (w593:T3)
          }
        }
        n256 = Select(t="Repeat?", s=w554, f="Longitudinal Profile") -> (s? t:f=w555:string)
      }
      frame "Repeat?" {
        # "Only reason to repeat is if TT Scheduling"
        n257 = local read "Task Selection"() -> (w604:T6)
        n258 = Unbundle By Name(w604) -> ("Turn Table Schedule"=w603:bool)
        n259 = case shown="False" w603 {
          tunnel: w611 -> [w614 w621]
          tunnel: [TRUE w620] -> w610
          tunnel: [w614 w619] -> w609
          tunnel: w605 -> [_ w618]
          frame False {
          }
          frame True {
            n260 = Array Size(array=w618) -> (size(s)=w617:i32)
            n261 = Decrement(x=w617) -> (x-1=w616:i32)
            n262 = in-place {
              in-place-border: w616 -> [w623]
              in-place-border: [w624] -> w620
              n263 = in-place-cluster #4(w621) -> ("Azimuth Array Index"=w622:u32)
              n264 = Equal?(x=w623, y=w622) -> (x = y?=w624:bool)
              n265 = case shown="True" w624 {
                tunnel: [w626 0] -> w625
                tunnel: w622 -> [w627 _]
                frame False {
                  n266 = Increment(x=w627) -> (x+1=w626:u32)
                }
                frame True {
                }
              }
              n267 = in-place-cluster #4("Azimuth Array Index"=w625) -> (w619:T16)
            }
          }
        }
        n268 = Select(t="End", s=w610, f="Zeroes" ("t")) -> (s? t:f=w606:string)
      }
      frame "End" {
        n269 = Unbundle By Name("Multirun Closure Tasks") -> ("Turn Table --> Zero"=w636:bool, "AutoCal"=w633:bool, "Zeroes"=w632:bool, "Global Cal Checks"=w631:bool, "Local Cal Checks"=w630:bool, "Tunnel Off"=w629:bool)
        n270 = while {
          shift-right: [w650] -> _
          shift-left: "Turn Table" -> [w651]
          tunnel: w636 -> [w649]
          tunnel: w633 -> [w646]
          tunnel: w632 -> [w645]
          tunnel: w631 -> [w644]
          tunnel: w630 -> [w643]
          tunnel: w629 -> [w642]
          shift-right: [w647] -> w634
          shift-left: w635 -> [w648]
          stop <- w641 continue-if-true
          n271 = case shown="\"Turn Table\"" w651 {
            tunnel: [_ "Zeroes" "AutoCal" "Global Cal Checks" "Local Cal Checks" "Tunnel Off" _] -> w650
            tunnel: w649 -> [_ w658 _ _ _ _ _]
            tunnel: w648 -> [w653 w657 w682 w706 w724 w745 w765]
            tunnel: [w653 w656 w681 w705 w723 w744 w764] -> w647
            tunnel: w646 -> [_ _ _ w703 _ _ _]
            tunnel: w645 -> [_ _ w679 _ _ _ _]
            tunnel: w644 -> [_ _ _ _ w721 _ _]
            tunnel: w643 -> [_ _ _ _ _ w742 _]
            tunnel: w642 -> [_ _ _ _ _ _ w763]
            tunnel: [FALSE TRUE TRUE TRUE TRUE TRUE TRUE] -> w641
            frame "No Match", Default {
            }
            frame "Turn Table" {
              n272 = case shown="True" w658 {
                tunnel: w657 -> [w659 w661]
                tunnel: [w659 w660] -> w656
                frame False {
                }
                frame True {
                  n273 = local read "Local Calcheck"() -> (w671:T8)
                  n274 = local read "Velocity (m/s)"() -> (w673:dbl)
                  n275 = Number To Fractional String(number=0.0) -> (F-format string=w665:string)  [unwired: 3 in]
                  n276 = Unbundle(w671) -> ("X"=w670:dbl, "Y"=w669:dbl, "Z"=w668:dbl, "Use Tunnel Coords? Coords"=w663:bool)  [unwired: 1 out]
                  n277 = case shown="True" w663 {
                    tunnel: ["" "!Work in Tunnel Coordinates"] -> w662
                    frame False {
                    }
                    frame True {
                    }
                  }
                  n278 = Concatenate Strings("MoveTT.vi;" ("Specific Arguments"), w665) -> (w666:string)
                  n279 = local read "RowTemplate"() -> (w674:T17)
                  n280 = Bundle By Name(cluster=w674, "Extra Commands"=w662, "Start X"=w670, "End X"=w670, "Start Y"=w669, "End Y"=w669, "Start Z"=w668, "End Z"=w668, "Tunnel Speed"=w673, "Row Type Selector"=Multi_run_mode."Run VI Named:", "Specific Arguments"=w666) -> (w664:T17)
                  n281 = Build Array (concatenate)(w661, w664) -> (w660:T3)
                }
              }
            }
            frame "Zeroes" {
              n282 = case shown="True" w679 {
                tunnel: w682 -> [w683 w685]
                tunnel: [w683 w684] -> w681
                frame False {
                }
                frame True {
                  n283 = local read "Results File Path / Name"() -> (w688:path)
                  n284 = local read "Measure (mins)"() -> (w689:dbl)
                  n285 = local read "Zeroes"() -> (w699:T7)
                  n286 = local read "Setup:"() -> (w691:string)
                  n287 = Unbundle(w699) -> ("X"=w695:dbl, "Y"=w694:dbl, "Z"=w693:dbl, "Use Tunnel Coords?"=w686:bool)  [unwired: 1 out]
                  n288 = case shown="False" w686 {
                    tunnel: ["" "!Work in Tunnel Coordinates"] -> w687
                    frame False {
                    }
                    frame True {
                    }
                  }
                  n289 = local read "RowTemplate"() -> (w698:T17)
                  n290 = Bundle By Name(cluster=w698, "Extra Commands"=w687, "Start X"=w695, "End X"=w695, "Start Y"=w694, "End Y"=w694, "Start Z"=w693, "End Z"=w693, "Meas Setup File"=w691, "Tunnel Speed"=0.0, "Comments"="Zeroes", "Row Type Selector"=Multi_run_mode."Single Measurement", "Averaging time (min)"=w689, "Filename"=w688) -> (w690:T17)
                  n291 = Build Array (concatenate)(w685, w690) -> (w684:T3)
                }
              }
            }
            frame "AutoCal" {
              n292 = case shown="True" w703 {
                tunnel: w706 -> [w707 w710]
                tunnel: [w707 w709] -> w705
                frame False {
                }
                frame True {
                  n293 = local read "Global Calcheck"() -> (w716:T7)
                  n294 = local read "Measure (mins)"() -> (w708:dbl)
                  n295 = local read "RowTemplate"() -> (w719:T17)
                  n296 = Unbundle(w716) -> ("X"=w715:dbl, "Y"=w714:dbl, "Z"=w713:dbl)  [unwired: 2 out]
                  n297 = Bundle By Name(cluster=w719, "Start X"=w715, "End X"=w715, "Start Y"=w714, "End Y"=w714, "Start Z"=w713, "End Z"=w713, "Averaging time (min)"=w708, "Comments"="AutoCalibrate", "Row Type Selector"=Multi_run_mode."Auto Calibrate", "Specific Arguments"="Tunnel Speed;2.18;3.06;4.37;5.68;7.86;10.26;13.1") -> (w711:T17)
                  n298 = Build Array (concatenate)(w710, w711) -> (w709:T3)
                }
              }
            }
            frame "Global Cal Checks" {
              n299 = case shown="True" w721 {
                tunnel: w724 -> [w725 w727]
                tunnel: [w725 w726] -> w723
                frame False {
                }
                frame True {
                  n300 = local read "Global Calcheck"() -> (w740:T7)
                  n301 = local read "Results File Path / Name"() -> (w731:path)
                  n302 = local read "Measure (mins)"() -> (w737:dbl)
                  n303 = local read "RowTemplate"() -> (w739:T17)
                  n304 = local read "Velocity (m/s)"() -> (w738:dbl)
                  n305 = local read "Setup:"() -> (w730:string)
                  n306 = Unbundle(w740) -> ("X"=w734:dbl, "Y"=w733:dbl, "Z"=w732:dbl)  [unwired: 2 out]
                  n307 = Bundle By Name(cluster=w739, "Start X"=w734, "End X"=w734, "Start Y"=w733, "End Y"=w733, "Start Z"=w732, "End Z"=w732, "Filename"=w731, "Tunnel Speed"=w738, "Comments"="CalCheck", "Row Type Selector"=Multi_run_mode."Single Measurement", "Averaging time (min)"=w737, "Meas Setup File"=w730, "Extra Commands"="!Work in Tunnel Coordinates") -> (w729:T17)
                  n308 = Build Array (concatenate)(w727, w729) -> (w726:T3)
                }
              }
            }
            frame "Local Cal Checks" {
              n309 = case shown="True" w742 {
                tunnel: w745 -> [w746 w748]
                tunnel: [w746 w747] -> w744
                frame False {
                }
                frame True {
                  n310 = local read "Local Calcheck"() -> (w761:T8)
                  n311 = local read "Results File Path / Name"() -> (w752:path)
                  n312 = local read "Measure (mins)"() -> (w758:dbl)
                  n313 = local read "RowTemplate"() -> (w760:T17)
                  n314 = local read "Velocity (m/s)"() -> (w759:dbl)
                  n315 = local read "Setup:"() -> (w751:string)
                  n316 = Unbundle(w761) -> ("X"=w755:dbl, "Y"=w754:dbl, "Z"=w753:dbl)  [unwired: 2 out]
                  n317 = Bundle By Name(cluster=w760, "Start X"=w755, "End X"=w755, "Start Y"=w754, "End Y"=w754, "Start Z"=w753, "End Z"=w753, "Filename"=w752, "Tunnel Speed"=w759, "Comments"="Local CalCheck", "Row Type Selector"=Multi_run_mode."Single Measurement", "Averaging time (min)"=w758, "Meas Setup File"=w751, "Extra Commands"="!Work in Tunnel Coordinates") -> (w750:T17)
                  n318 = Build Array (concatenate)(w748, w750) -> (w747:T3)
                }
              }
            }
            frame "Tunnel Off" {
              n319 = case shown="True" w763 {
                tunnel: w765 -> [w766 w777]
                tunnel: [w766 w776] -> w764
                frame False {
                }
                frame True {
                  n320 = local read "Global Calcheck"() -> (w772:T7)
                  n321 = local read "RowTemplate"() -> (w775:T17)
                  n322 = Unbundle(w772) -> ("X"=w771:dbl, "Y"=w770:dbl, "Z"=w769:dbl)  [unwired: 2 out]
                  n323 = Bundle By Name(cluster=w775, "Start X"=w771, "End X"=w771, "Start Y"=w770, "End Y"=w770, "Start Z"=w769, "End Z"=w769, "Tunnel Speed"=0.0, "Comments"="Tunnel Off", "Row Type Selector"=Multi_run_mode."Set Tunnel Speed Only") -> (w768:T17)
                  n324 = Build Array (concatenate)(w777, w768) -> (w776:T3)
                }
              }
            }
          }
        }
      }
    }
    n325 = Or(x=w19, y="Stop Button") -> (x .or. y?=w18:bool)
    n326 = local write "Index Tracking"(w17) -> ()
  }
  "Audit Array" <- w6
  n327 = local write "TaskArray"(w1) -> ()
  n328 = local write "Index Tracking"(w5) -> ()
  n329 = local read "Task Selection"() -> (w2:T6)
  n330 = Unbundle By Name(w2) -> ("Save Command File"=w3:bool)
  n331 = case shown="True" w3 {
    tunnel: "Command File Path / Name" -> [_ w780]
    tunnel: w1 -> [_ w778]
    frame False {
    }
    frame True {
      n332 = call "Multi_Run_Prog.vi"("Command filename"=w780, "Mode"=T23."Save Command File", "Table"=w778) -> ()  [unwired: 17 in]
    }
  }
